vi "Robot Polish Demo.vi"() -> ()   [LabVIEW 2016]
uses:
  <vilib>/Platform/TimedLoop/XDataNode/timing_clust.ctl
  <vilib>/Platform/TimedLoop/XDataNode/nitl_modes.ctl
  <vilib>/Platform/TimedLoop/XDataNode/wakeup.ctl
  Subsystems/Global Variables.vi
  <vilib>/FPGAPlugInAG/PXI-7833R/niLvFpga_Open_PXI-7833R.vi
  <vilib>/Utility/error.llb/Error Cluster From Error Code.vi
  <vilib>/rvi/errors/niLvFpgaAdjustHostInterfaceError.vi
  <vilib>/Utility/file.llb/Write Delimited Spreadsheet (string).vi
  <vilib>/Utility/file.llb/Write Delimited Spreadsheet (DBL).vi
  <vilib>/FPGAPlugInAG/PXI-7833R/niLvFpga_Reset_PXI-7833R.vi
  <vilib>/FPGAPlugInAG/PXI-7833R/niLvFpga_Close_PXI-7833R.vi
  <vilib>/rvi/interface/nirviOpenFPGA/nirviOpenFPGA.xnode
  FPGA Bitfiles/PhantomControlPI_FPGATarget_QuadCtr2_E2412E44.lvbitx
  IRISS_FPGA_IO.vi
  <vilib>/rvi/interface/nirviReadWriteControl/nirviReadWriteControl.xnode
  <vilib>/platform/TimedLoop/XDataNode/XDataNode.xnode
  <vilib>/rvi/interface/nirviMethod/nirviMethod.xnode
  <vilib>/rvi/interface/nirviCloseFPGA/nirviCloseFPGA.xnode
  Library/KevinLibraryAll/labview2011/kevLib2011.lvlib
  NiFpgaLv.dll
  <vilib>/Platform/TimedLoop/XDataNode/XDNodeRunTimeDep.lvlib
panel:
  in  "OCT Z":dbl
  out "Current Iter. No.":u16
  in  "Set Iter. No.":i32=5
  in  "Learning Type":enum8{"Cyber Learning", "Physical Learning"}(ring)=enum."Physical Learning"
  out "RUY Cluster":T1
  in  "Pause":bool caption="To M/S"
  in  "No. Cycles":u8=1
  in  "L4 [deg]":dbl
  in  "L3 [mm]":dbl step=0.1
  in  "L2 [deg]":dbl
  in  "L1 [deg]":dbl
  out "Trajectory Cluster":T2
  out "Update Mdl & Traj":bool=TRUE
  out "Stage PID Cluster":T3={"Stage Z PID"={"Kp"=0.0005, "Kd"=0.001, "Ki"=0.0}, "Stage Y PID"={"Kp"=0.0003, "Kd"=0.01, "Ki"=0.0}, "Stage X PID"={"Kp"=0.0003, "Kd"=0.01, "Ki"=0.0}}
  out "L1 to L4 PID Cluster":T4={"L1 PID Gains"={"Kp"=0.005, "Kd"=0.5, "Ki"=0.0005}, "L2 PID Gains"={"Kp"=0.01, "Kd"=1.0, "Ki"=0.0005}, "L3 PID Gains"={"Kp"=0.05, "Kd"=1.0, "Ki"=0.0005}, "L4 PID Gains"={"Kp"=0.1, "Kd"=1.0, "Ki"=0.0005}}
  in  "IRISS GUI":T5(tab)
  in  "OCT Home Dir":bool
  out "X Stage out [mm] 2":dbl caption="Stage X [mm]" format="%#.4f"
  out "Z Stage out [mm] 2":dbl caption="Stage Z [mm]" format="%#.4f"
  out "Y Stage out [mm] 2":dbl caption="Stage Y [mm]" format="%#.4f"
  out "Vacuum Force [mmHg]  2":i32 caption="[mmHg]"
  out "Finished Late Counts":u16
  out "Emergency alarm":bool
  out "Remote sender engaged":bool
  in  "L2 PID Gains":cluster{"Kp":dbl, "Kd":dbl, "Ki":dbl}={"Kp"=0.01, "Kd"=1.0, "Ki"=0.005}
  in  "L3 PID Gains":cluster{"Kp":dbl, "Kd":dbl, "Ki":dbl}={"Kp"=0.05, "Kd"=1.0, "Ki"=0.0005}
  in  "L4 PID Gains":cluster{"Kp":dbl, "Kd":dbl, "Ki":dbl}={"Kp"=0.1, "Kd"=0.1, "Ki"=0.0005}
  in  "L1 PID Gains":cluster{"Kp":dbl, "Kd":dbl, "Ki":dbl}={"Kp"=0.01, "Kd"=0.5, "Ki"=0.001}
  out "Current System State":T6(ring)
  out "State changing":bool
  out "Tip out Posit":dbl[](array[numeric]) caption="Position [mm]" format="%#.3f"
  out "Tip cmd Posit":dbl[](array[numeric]) caption="Command [mm]" format="%#.3f"
  out "L4 out Posit":dbl caption="y [deg]" format="%#.2g"
  out "L4 cmd Posit":dbl caption="r [deg]" format="%#.2g"
  out "L3 out Posit":dbl caption="y [mm]" format="%#.2g"
  out "L3 cmd Posit":dbl caption="r [mm]" format="%#.2g"
  out "L2 out Posit":dbl caption="y [deg]" format="%#.2g"
  out "L2 cmd Posit":dbl caption="r [deg]" format="%#.2g"
  out "L1 out Posit":dbl caption="y [deg]" format="%#.2g"
  out "L1 cmd Posit":dbl caption="r [deg]" format="%#.2g"
  out "State Flag Array":bool[](array[boolean])
  out "Irrigation Engaged? 2":bool caption="Irrigation Engaged"
  out "Task Space Error":dbl[][](graph)
  in  "Learning Gains":dbl[](array[numeric])=[0.75, 1.0, 0.75, 0.0]
  in  "Joint Limits":dbl[][](array[numeric])=[[-8.0, 50.0], [-35.0, 35.0], [-5.0, 20.0], [-180.0, 180.0]] format="%#.3g"
  out "First Trk Pt":dbl[](array[numeric]) format="%#.3g"
  in  "Offset Home 2 RCM":dbl[](array[numeric])=[-7.7, 37.0, 55.0, 0.0] format="%#.3g"
  out "Error(s) Out on Program End":errorcluster
  out "L4 Chart":dbl(graph)
  out "L3 Chart":dbl(graph)
  out "L2 Chart":dbl(graph)
  out "L1 Chart":dbl(graph)
  out "L1 Tracking":dbl[][](graph)
  out "L2 Tracking":dbl[][](graph)
  out "L3 Tracking":dbl[][](graph)
  out "L4 Tracking":dbl[][](graph)
  out "L1 Cmd":dbl[](graph)
  out "L2 Cmd":dbl[](graph)
  out "L4 Cmd":dbl[](graph)
  out "L3 Cmd":dbl[](graph)
  in  "Clear Charts":bool
  out "AC Pressure [mmHg]":sgl
  in  "Irrigation?":bool
  in  "PID ON/OFF":bool
  in  "Vac PID Gains":cluster{"Kp":dbl, "Kd":dbl, "Ki":dbl, "Ts":dbl}={"Kp"=5.0, "Kd"=0.0, "Ki"=5.0, "Ts"=0.01}
  in  "Vac Cmd":sgl min=0 max=100 step=1 format="%#_13g"
  in  "Target IOP":sgl=20.0 min=0 max=100 step=1 format="%#_13g"
  out "IOP Ctrl":T7(graph)
  out "Pressure Sensors":T8(graph)
  in  "Remote Control Source":u16(ring) caption="Remote Source" items=["Surgical Console", "Joystick"]
  in  "Reset Joystick":bool caption="Encoder Reset"
  in  "Max Limit [mmHg]":dbl=600.0
  out "Pressure Reading":dbl[](array[numeric]) caption="IOP Output [mmHg]"
  in  "Hydration":bool
  out "Vac Input":sgl
  in  "Wait Time [ms]":i32=200
  in  "Vac Step Size":sgl=50.0 min=0 max=100 step=1 format="%#_13g"
  in  "Increase":bool
  in  "Vacuum Step":bool
  in  "Take IOP Data":bool
  out "Elaspsed Time":sgl
  in  "Seconds of Data":sgl=5.0
  out "File Exists":bool
  out "File Path":path=path "C:/IOPData1.txt"
  in  "Data No":i16=1 min=1 step=1
  in  "Eye No":i16=1 min=1 step=1
  out "OCT Z out [mm]":dbl caption="OCT Out Z [mm]" format="%#.4f"
  out "OCT Z cmd [mm]":dbl=6.0 caption="OCT Z Ref [mm]" min=0.0 max=12.0 step=0.5
  in  "OCT Z PID Gains":cluster{"Kp":dbl, "Kd":dbl, "Ki":dbl}={"Kp"=0.0003, "Kd"=0.0001, "Ki"=0.01}
  out "Z Stage out [mm]":dbl caption="Output Z [mm]" format="%#.4f"
  out "Z Stage cmd [mm]":dbl=6.0 caption="Reference Z [mm]" min=0.0 max=12.0 step=0.5
  out "Y Stage out [mm]":dbl caption="Output Y [mm]" format="%#.4f"
  out "Y Stage cmd [mm]":dbl=6.0 caption="Reference Y  [mm]" min=0.0 max=12.0 step=0.5
  out "X Stage out [mm]":dbl caption="Output X [mm]" format="%#.4f"
  out "X Stage cmd [mm]":dbl=6.0 caption="Reference X [mm]" min=0.0 max=12.0 step=0.5
  in  "Stage Z PID Gains":cluster{"Kp":dbl, "Kd":dbl, "Ki":dbl}={"Kp"=0.0005, "Kd"=0.001, "Ki"=0.0}
  in  "Stage Y PID Gains":cluster{"Kp":dbl, "Kd":dbl, "Ki":dbl}={"Kp"=0.0001, "Kd"=0.005, "Ki"=0.0}
  in  "Stage X PID Gains":cluster{"Kp":dbl, "Kd":dbl, "Ki":dbl}={"Kp"=0.0003, "Kd"=0.01, "Ki"=0.0}
  out "Irrigation Engaged?":bool
  out "Accurus Button":bool[](array[boolean]) caption="Remote Button Command"
  in  "Control: Vacuum Force":i8(slide) min=0 max=78 step=1 scale=0.0..78.0
  out "Voltage Output Ch. B":dbl(graph)
  out "Voltage Output Ch. A":dbl(graph)
  out "Accurus Engaged?":bool
  out "Vacuum Force [mmHg]":i32
  in  "Load Traj":bool caption="To M/S"
  in  "Retract":bool caption="To M/S"
  in  "Stop Accurus":bool caption="To M/S"
  in  "L3 Go Home":bool caption="To M/S"
  in  "Track":bool caption="To M/S"
  in  "Program Stop":bool
  in  "Iterate":bool caption="To M/S"
  # "Track Params"
  # "ILC Params"
  # "Tool Tip Location"
  # "L1"
  # "Robot Status"
  # "X\nY\nZ"
  # "X\nY\nZ"
  # "L2"
  # "System Progress"
  # "L3"
  # "Homing finished"
  # "Task Space Error"
  # "M/S initialization finished"
  # "Trajecoty loading finished"
  # "Tracking initialization finished"
  # "L4"
  # "In Tracking"
  # "Notes: \n2. check state transition\n4. preview trajectory?"
  # "Vacuum"
  # "Calibration"
  # "Space Deform Parameters"
  # "Joint Motion"
  # "S"
  # "L1"
  # "[deg]"
  # "R"
  # "[deg]"
  # "L2"
  # "[deg]"
  # "T"
  # "[mm]"
  # "L3"
  # "[mm]"
  # "L4"
  # "[deg]"
  # "AC & PC Gap"
  # "First Track Point"
  # "L1"
  # "[deg]"
  # "L2"
  # "[deg]"
  # "L3"
  # "[mm]"
  # "L4"
  # "[deg]"
  # "Tracking Joint Limits"
  # "Error Message"
  # "Incision"
  # "Min."
  # "Max."
  # "L1"
  # "L1"
  # "[deg]"
  # "L2"
  # "L2"
  # "[deg]"
  # "L3"
  # "L3"
  # "[mm]"
  # "L4"
  # "L4"
  # "[deg]"
  # "IOP Feedback Control"
  # "Data Saving"
  # "Vacuum Step"
  # "XYZ Stage Control"
  # "OCT Z-Axis"
  # "Foot Pedal Buttons"
  # "Irrigation and Aspiration"
  # "Button 1"
  # "Button 2"
  # "Button 3"
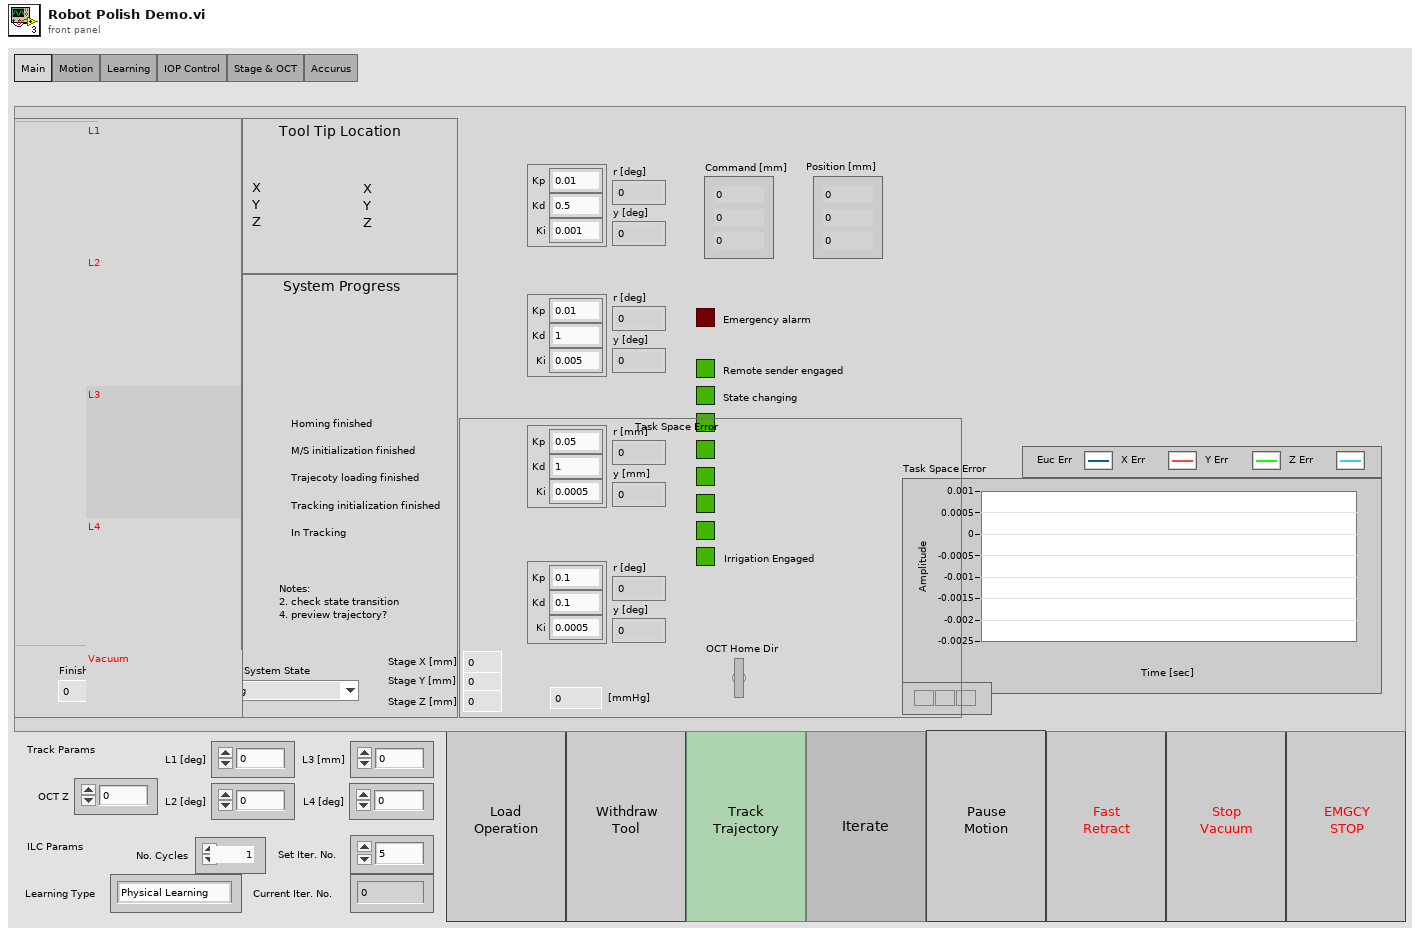
[diagram p1: front panel]
types:
  T1 = cluster{"Ref":cluster{"theta 1 Array":dbl[], "theta 2 Array":dbl[], "d3 Array":dbl[], "theta 4 Array":dbl[]}, "uFF":cluster{"theta 1 Array":dbl[], "theta 2 Array":dbl[], "d3 Array":dbl[], "theta 4 Array":dbl[]}, "yOut":cluster{"theta 1 Array":dbl[], "theta 2 Array":dbl[], "d3 Array":dbl[], "theta 4 Array":dbl[]}}
  T2 = cluster{"Traj Px Array":dbl[], "Traj Py Array":dbl[], "Traj Pz Array":dbl[]}
  T3 = cluster{"Stage Z PID":cluster{"Kp":dbl, "Kd":dbl, "Ki":dbl}, "Stage Y PID":cluster{"Kp":dbl, "Kd":dbl, "Ki":dbl}, "Stage X PID":cluster{"Kp":dbl, "Kd":dbl, "Ki":dbl}}
  T4 = cluster{"L1 PID Gains":cluster{"Kp":dbl, "Kd":dbl, "Ki":dbl}, "L2 PID Gains":cluster{"Kp":dbl, "Kd":dbl, "Ki":dbl}, "L3 PID Gains":cluster{"Kp":dbl, "Kd":dbl, "Ki":dbl}, "L4 PID Gains":cluster{"Kp":dbl, "Kd":dbl, "Ki":dbl}}
  T5 = enum32{"Main", "Motion", "Learning", "IOP Control", "Stage & OCT", "Accurus"}
  T6 = enum16{"Homing", "M/S Initialization", "M/S Operation", "Trajectory Loading", "Tracking Initialization", "Tracking", "Physical Learning", "Cyber Learning"}
  T7 = cluster{"[0]":sgl, "[1]":sgl, "[2]":sgl, "[3]":sgl, "[4]":sgl, "[5]":sgl, "[6]":sgl, "[7]":sgl, "[8]":sgl}
  T8 = cluster{"pressure sensors[0]":sgl, "pressure sensors[1]":sgl, "pressure sensors[2]":sgl, "pressure sensors[3]":sgl, "pressure sensors[4]":sgl, "pressure sensors[5]":sgl, "pressure sensors[6]":sgl, "pressure sensors[7]":sgl, "pressure sensors[8]":sgl}
  T9 = cluster{"theta 1 Array":dbl[], "theta 2 Array":dbl[], "d3 Array":dbl[], "theta 4 Array":dbl[]}
  T10 = cluster{"Prev L1 to L4 Posit":dbl[], "Prev Stage Posit":dbl[], "Prev OCT Z Posit":dbl}
  T11 = typedef "XDNodeRunTimeDep.lvlib/timing_clust.ctl" = cluster{"Expected End [f-1]":u64, "Actual End [f-1]":u64, "Finished Late? [f-1]":bool, "Expected End [i-1]":u64, "Actual End [i-1]":u64, "Finished Late? [i-1]":bool, "Expected Start [i]":u64, "Actual Start [i]":u64, "Expected Start [f]":u64, "Actual Start [f]":u64, "Source Name":string, "Structure Name":string, "Period":i64, "Deadline":i64, "Offset":i64, "Start":i64, "Priority":i32, "Timeout":i32, "Mode":T12, "Wakeup Reason":T13, "Error":errorcluster, "Source Type":string, "Secondary Source Type":string, "Global End Time":u64, "Global Start Time":u64, "Frame Duration":u64, "Iteration Duration":u64, "Assigned CPU":i32, "I/O Scan Engine Mode":u32}
  T12 = typedef "XDNodeRunTimeDep.lvlib/nitl_modes.ctl" = enum32{"No Change", "Process missed periods, maintain original phase", "Discard missed periods, maintain original phase", "Process missed periods, ignore original phase", "Discard missed periods, ignore original phase"}
  T13 = typedef "XDNodeRunTimeDep.lvlib/wakeup.ctl" = enum32{"Normal", "Aborted", "Asynchronous wakeup", "Timing source error", "Timed loop error", "Timeout"}
  T14 = cluster{"L1 to L4 PID Cluster":cluster{"L1 PID Gains":cluster{"Kp":dbl, "Kd":dbl, "Ki":dbl}, "L2 PID Gains":cluster{"Kp":dbl, "Kd":dbl, "Ki":dbl}, "L3 PID Gains":cluster{"Kp":dbl, "Kd":dbl, "Ki":dbl}, "L4 PID Gains":cluster{"Kp":dbl, "Kd":dbl, "Ki":dbl}}, "Stage PID Cluster":cluster{"Stage Z PID":cluster{"Kp":dbl, "Kd":dbl, "Ki":dbl}, "Stage Y PID":cluster{"Kp":dbl, "Kd":dbl, "Ki":dbl}, "Stage X PID":cluster{"Kp":dbl, "Kd":dbl, "Ki":dbl}}, "OCT Z PID Gains":cluster{"Kp":dbl, "Kd":dbl, "Ki":dbl}}
  T15 = enum8{"Enabled", "Disabled", "Disabled and Grayed Out"}
  T16 = cluster{"Accurus button":bool[], "Accurus engaged?":bool, "Vacuum Force":i32, "Accurus Ch. A Vout":dbl, "Accurus Ch. B Vout":dbl, "Irrigation engaged?":bool}
  T17 = cluster{"pressure sensors[0]":sgl, "pressure sensors[1]":sgl, "pressure sensors[2]":sgl, "pressure sensors[3]":sgl, "pressure sensors[4]":sgl, "pressure sensors[5]":sgl, "pressure sensors[6]":sgl, "pressure sensors[7]":sgl, "pressure sensors[8]":sgl}[]
  T18 = cluster{"Last L1 to L4 Posit":dbl[], "Last Stage Posit":dbl[], "Last OCT Z Posit":dbl}
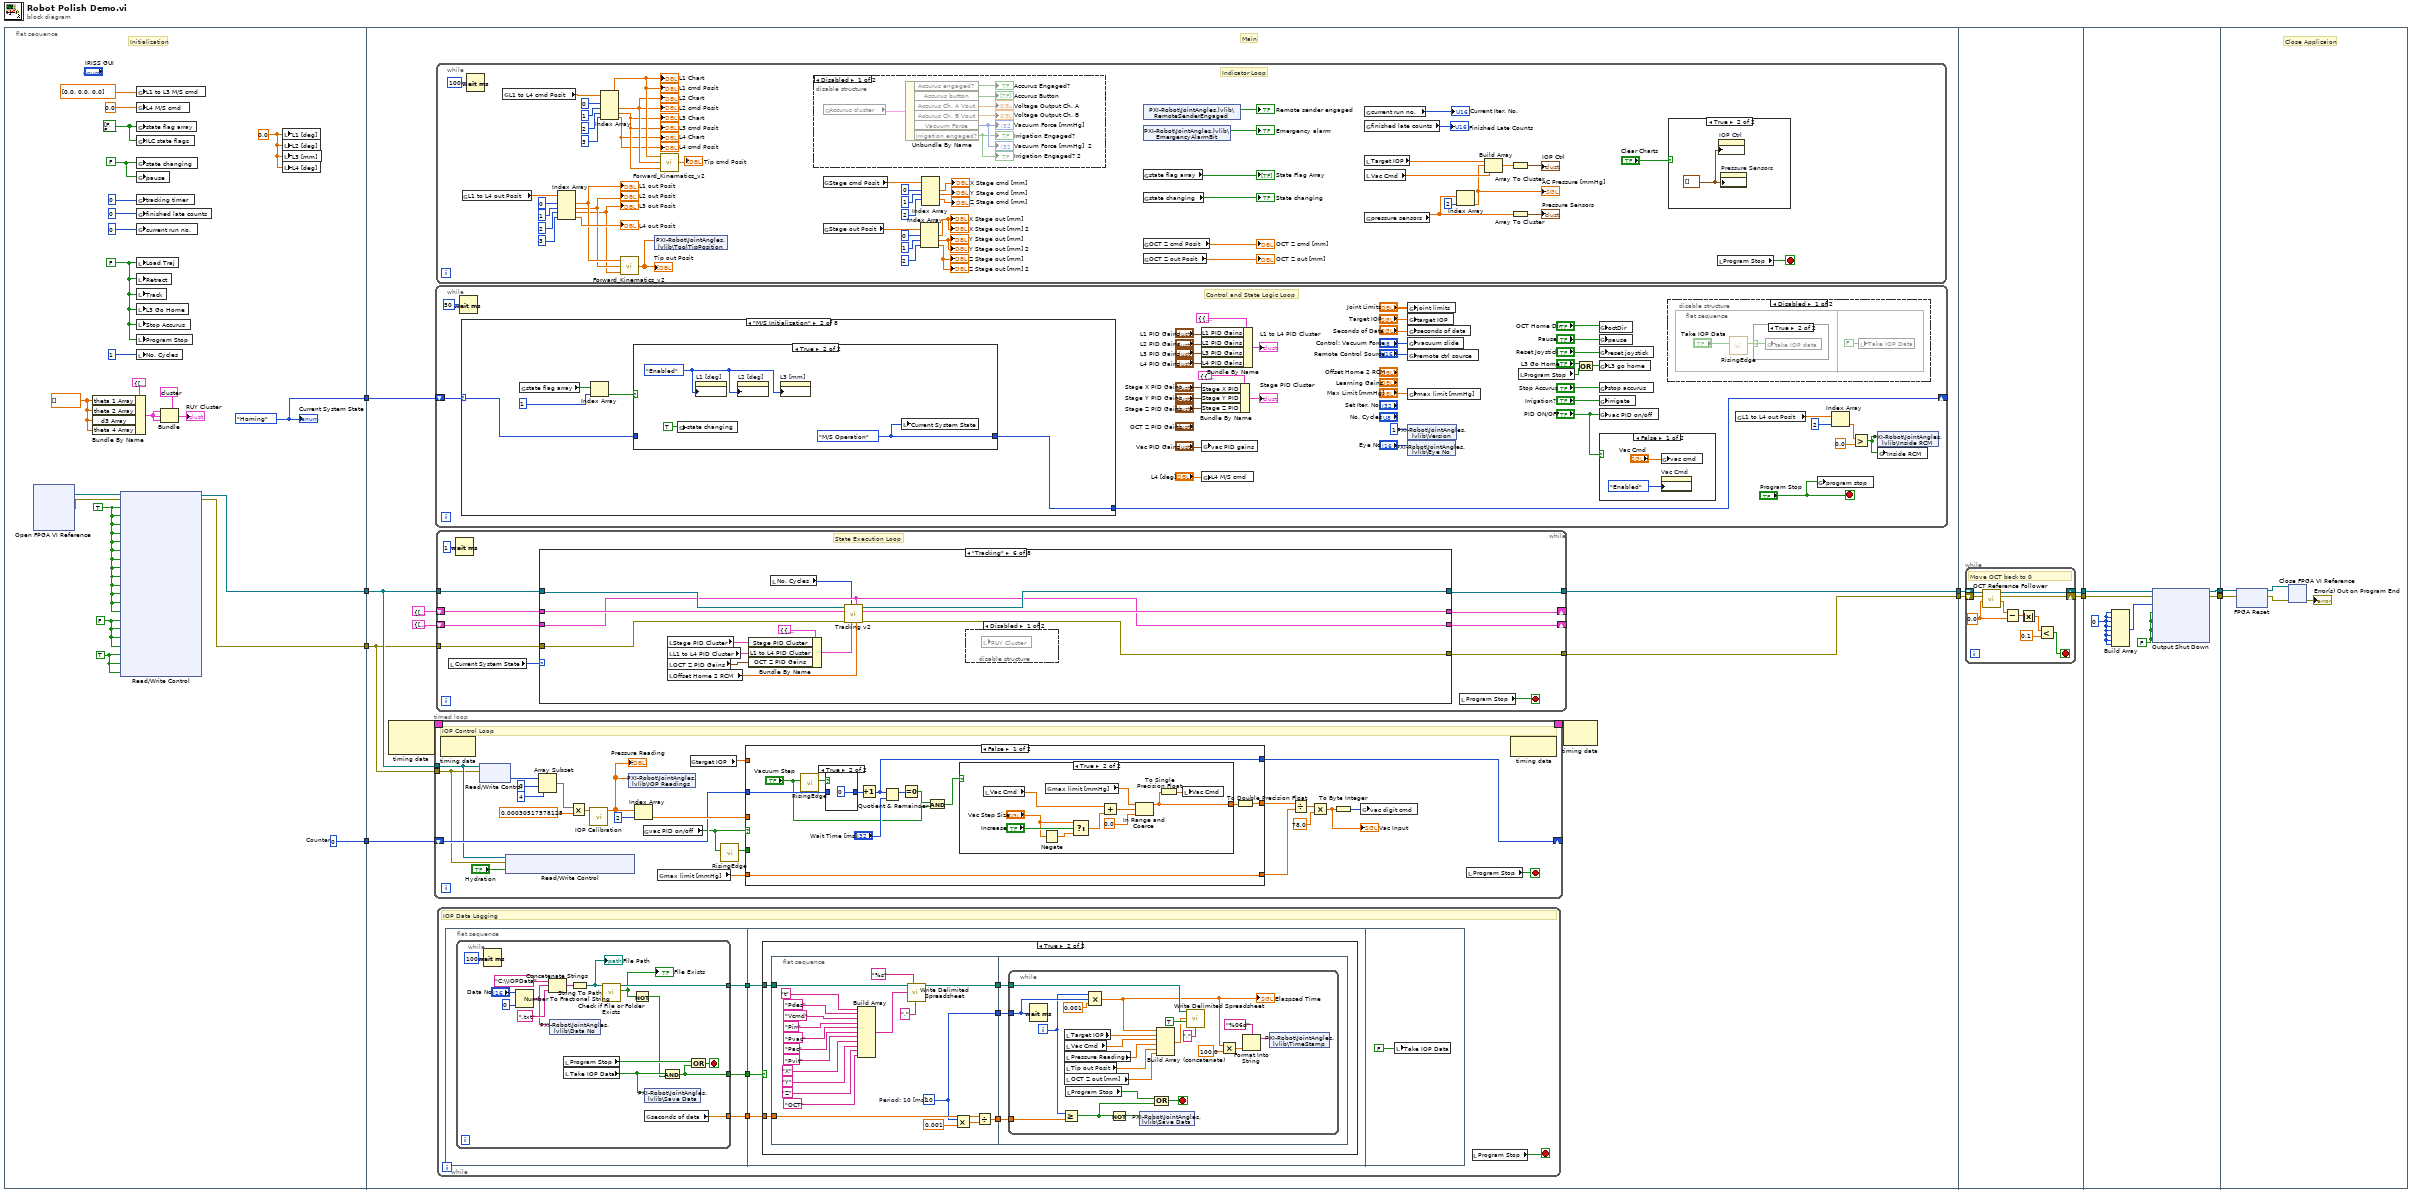
[diagram p0: block diagram]
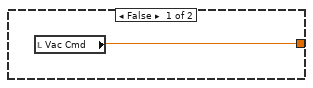
[diagram p4: hidden frame]
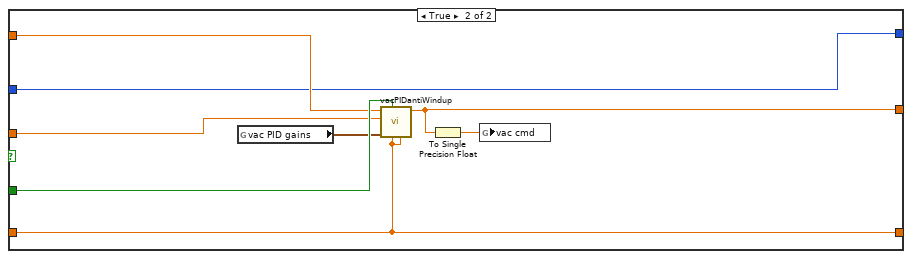
[diagram p5: hidden frame]
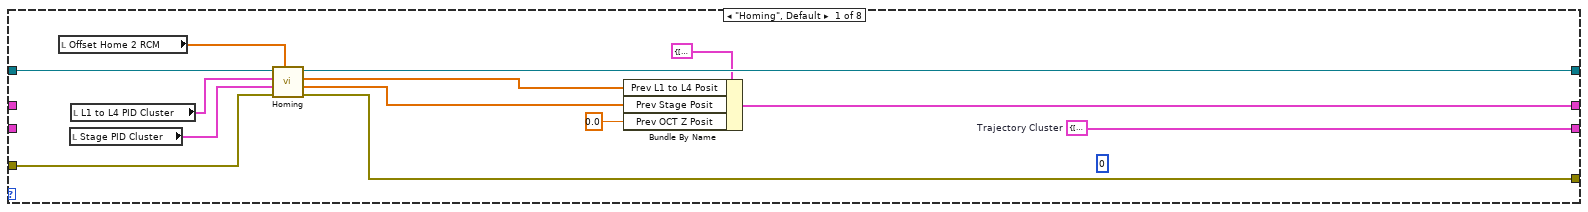
[diagram p8: hidden frame]
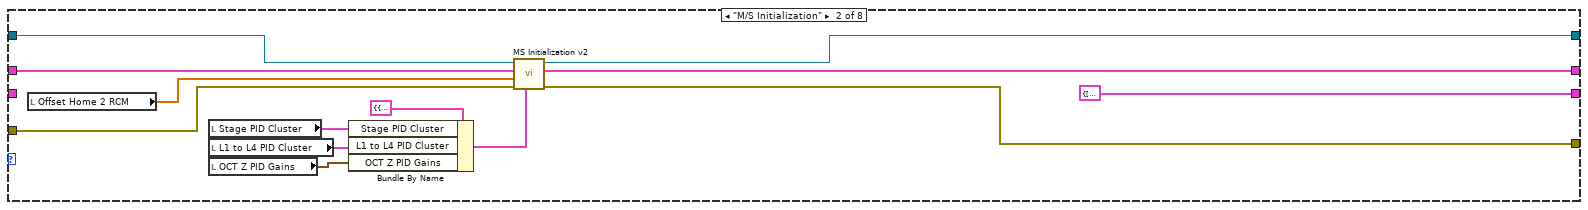
[diagram p9: hidden frame]
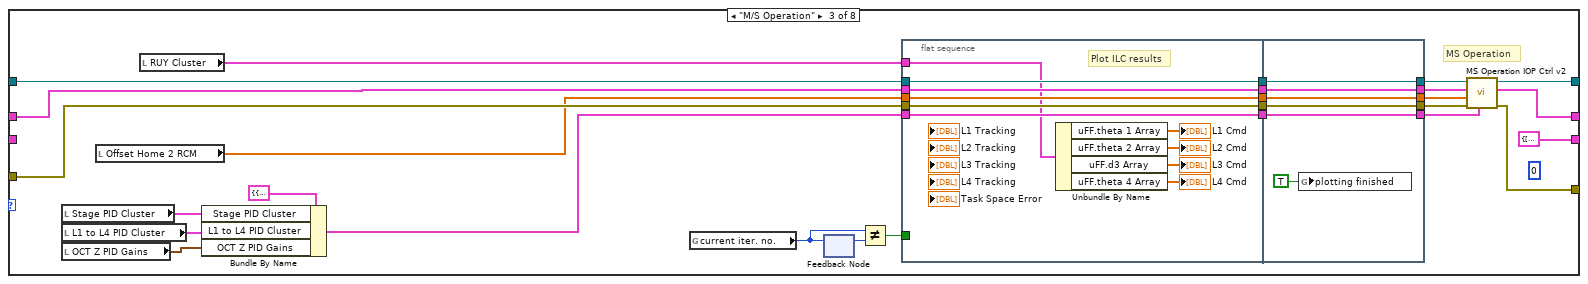
[diagram p10: hidden frame]
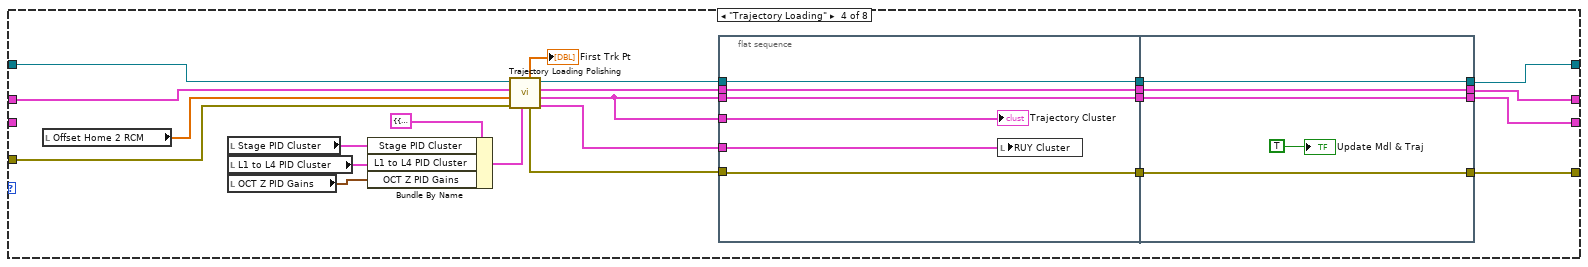
[diagram p11: hidden frame]
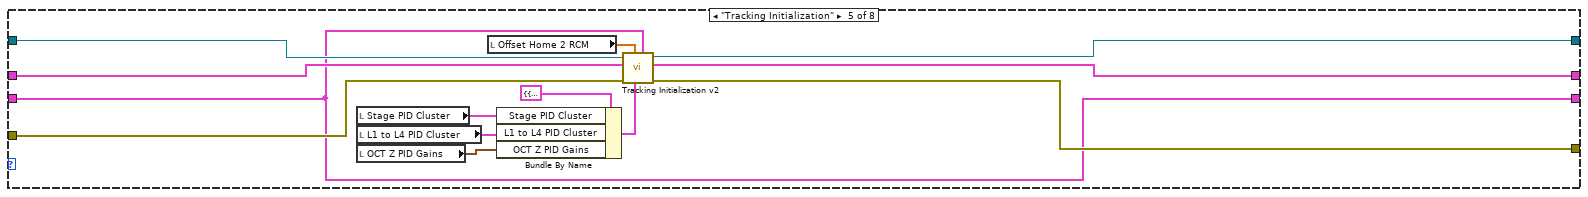
[diagram p12: hidden frame]
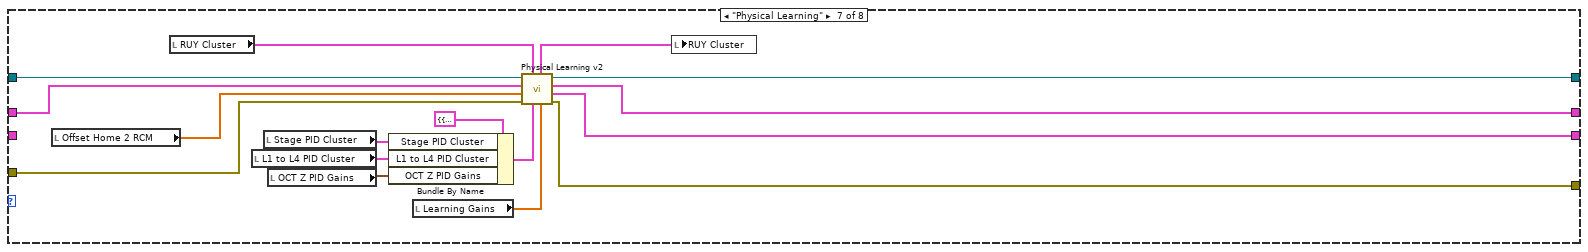
[diagram p14: hidden frame]
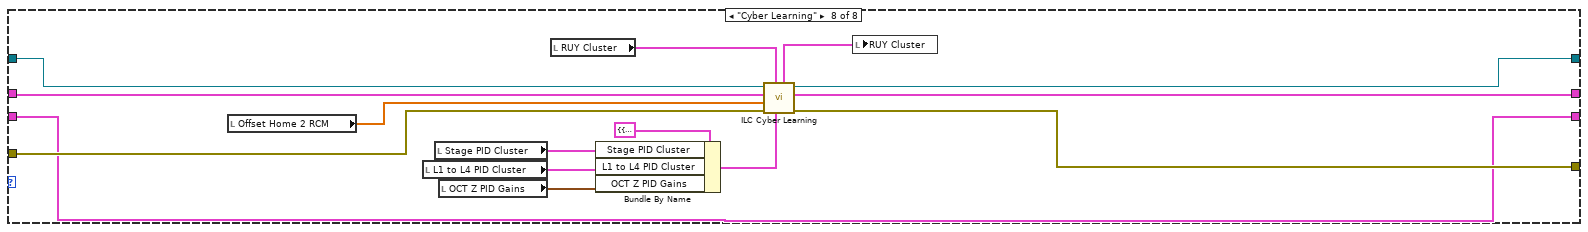
[diagram p15: hidden frame]
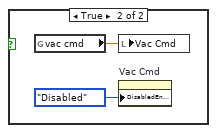
[diagram p18: hidden frame]
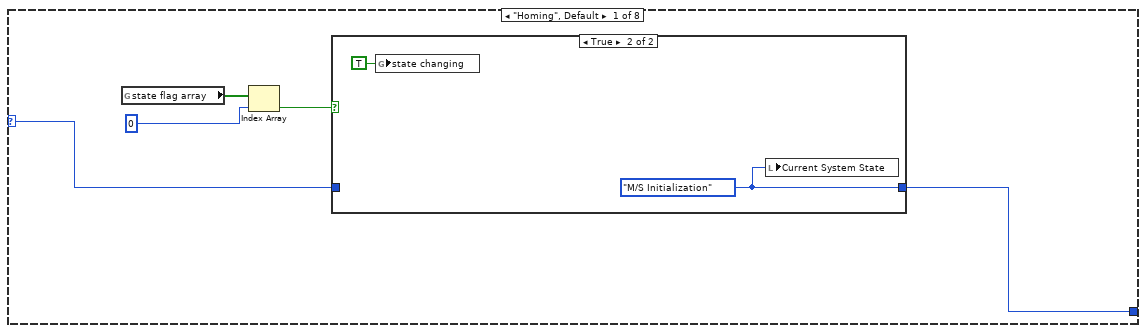
[diagram p19: hidden frame]
diagram:
  n1 = flat-sequence {
    tunnel: [w29] -> w10
    tunnel: [w28] -> w9
    tunnel: [w24] -> w8
    tunnel: [w11] -> w7
    tunnel: w7 -> [w38]
    tunnel: w8 -> [w41]
    tunnel: w9 -> [w39]
    tunnel: w10 -> [w37]
    tunnel: [w36] -> w4
    tunnel: [w35] -> w2
    tunnel: w4 -> [w608]
    tunnel: [w610] -> w3
    tunnel: w2 -> [w609]
    tunnel: [w611] -> w1
    tunnel: [w625] -> w6
    tunnel: [w624] -> w5
    tunnel: w3 -> [w622]
    tunnel: w1 -> [w623]
    tunnel: w6 -> [w630]
    tunnel: w5 -> [w629]
    frame #0 {
      w11 = 0  # Counter
      w12 = dbl[] [] ("theta 1 Array")
      w18 = 0.0 ("L4 M/S cmd")
      w24 = T6."Homing" ("Current State")
      w17 = bool[] [FALSE, FALSE, FALSE, FALSE, FALSE, FALSE, FALSE, FALSE, FALSE] ("state flag array")
      w25 = FALSE ("state changing")
      w33 = TRUE ("Conn0/DIO12 Button 1")
      w32 = FALSE ("Reset")
      w34 = TRUE ("Reset")
      w26 = FALSE ("program stop")
      # "Initialization"
      n2 = xnode "Open FPGA VI Reference"() -> ("FPGA VI Reference Out"=w31:refnum<k20>, "error out"=w30:errorcluster)  [unwired: 2 in]
      n3 = Bundle By Name(cluster=T9 {"theta 1 Array"=[], "theta 2 Array"=[], "d3 Array"=[], "theta 4 Array"=[]} ("uFF"), "theta 1 Array"=w12, "theta 2 Array"=w12, "d3 Array"=w12, "theta 4 Array"=w12) -> (w13:T9)
      n4 = xnode "Read/Write Control"("FPGA VI Reference In"=w31, "error in"=w30, "Reset 1"=w34, "Reset 3"=w34, "Reset 9"=w34, "Reset 10"=w34, "Reset 11"=w34, "Reset 12"=w34, "Reset 13"=w34, "Reset 14"=w34, "Reset 15"=w34, "Reset 16"=w34, "Reset 17"=w34, "Reset C1-1"=w34, "Reset C1-4"=w34, "INHB X"=w32, "INHB Y"=w32, "INHB Z"=w32, "INHB OCT Mot"=w32, "Conn0/DIO12 Button 1"=w33, "Conn0/DIO13 Button 2"=w33, "Conn0/DIO15 Button 4"=w33) -> ("FPGA VI Reference Out"=w28:refnum<k20>, "error out"=w29:errorcluster)
      n5 = global write "Global Variables.vi" "L1 to L3 M/S cmd"(dbl[] [0.0, 0.0, 0.0] ("L1 to L3 M/S cmd")) -> ()
      n6 = global write "Global Variables.vi" "L4 M/S cmd"(0.0 ("L4 M/S cmd")) -> ()
      n7 = global write "Global Variables.vi" "state flag array"(w17) -> ()
      n8 = global write "Global Variables.vi" "ILC state flags"(w17) -> ()
      n9 = global write "Global Variables.vi" "state changing"(w25) -> ()
      n10 = global write "Global Variables.vi" "pause"(w25) -> ()
      n11 = global write "Global Variables.vi" "tracking timer"(0 ("finished late counts")) -> ()
      n12 = global write "Global Variables.vi" "finished late counts"(u16 0 ("finished late counts")) -> ()
      n13 = global write "Global Variables.vi" "current run no."(u8 0 ("current run no.")) -> ()
      n14 = local write "Load Traj"(w26) -> ()
      n15 = local write "Retract"(w26) -> ()
      n16 = local write "Track"(w26) -> ()
      n17 = local write "L3 Go Home"(w26) -> ()
      n18 = local write "Stop Accurus"(w26) -> ()
      n19 = local write "Program Stop"(w26) -> ()
      n20 = local write "No. Cycles"(1 ("No. Cycles")) -> ()
      n21 = Bundle(cluster=T1 {"Ref"={"theta 1 Array"=array[6000 elements], "theta 2 Array"=array[6000 elements], "d3 Array"=array[6000 elements], "theta 4 Array"=array[6000 elements]}, "uFF"={"theta 1 Array"=array[6000 elements], "theta 2 Array"=array[6000 elements], "d3 Array"=array[6000 elements], "theta 4 Array"=array[6000 elements]}, "yOut"={"theta 1 Array"=[], "theta 2 Array"=[], "d3 Array"=[], "theta 4 Array"=[]}} ("Cluster"), "Ref"=w13, "uFF"=w13, "yOut"=w13) -> (→"RUY Cluster":T1)
      n22 = local write "L1 [deg]"(w18) -> ()
      n23 = local write "L2 [deg]"(w18) -> ()
      n24 = local write "L3 [mm]"(w18) -> ()
      n25 = local write "L4 [deg]"(w18) -> ()
      "Current System State" <- w24
    }
    frame #1 {
      # "Main"
      n26 = node-c288 ("Input Node")() -> (w44:T11)  [unwired: 2 in]
      n27 = timed-loop {
        timing: w44 -> [_]
        timing-out: [_] -> w43
        tunnel: w39 -> [w129]
        tunnel: w37 -> [w128]
        shift-right: [w130] -> _
        shift-left: w38 -> [w131]
        stop <- w139 stop-if-true
        # "IOP Control Loop"
        n28 = node-c288() -> ()  [unwired: 1 in, 1 out]
        n29 = xnode "Read/Write Control"("FPGA VI Reference In"=w129, "error in"=w128) -> ("AI"=w142:i16[])  [unwired: 2 out]
        n30 = xnode "Read/Write Control"("FPGA VI Reference In"=w129, "error in"=w128, "Hydration On/Off (Connector2/DIO28)"="Hydration") -> ()  [unwired: 2 out]
        n31 = Array Subset(array=w142, index=0, length=4) -> (w147:i16[])
        n32 = Multiply(x=w147, y=0.00030517578125) -> (x*y=w134:dbl[])
        n33 = call "IOP Calibration.vi"("IOP Input [V]"=w134) -> ("IOP Output [mmHg]"=w123:dbl[])  [unwired: 10 in]
        "Pressure Reading" <- w123
        n34 = shared-variable "PXI-Robot\\JointAngles.lvlib\\IOP Readings"(w123) -> ()  [unwired: 1 in, 1 out]
        n35 = Index Array(array=w123, index=2) -> (element=w140:dbl)
        n36 = global read "Global Variables.vi" "vac PID on/off"() -> (w124:bool)
        n37 = global read "Global Variables.vi" "max limit [mmHg]"() -> (w125:dbl)
        n38 = global read "Global Variables.vi" "target IOP"() -> (w126:sgl)
        n39 = call "RisingEdge.vi"("Signal In"=w124) -> ("Rising Edge"=w141:bool)  [unwired: 10 in]
        n40 = case shown="False" w124 {
          tunnel: w140 -> [_ w176]
          tunnel: w126 -> [_ w177]
          tunnel: [w159 w180] -> w138
          tunnel: w125 -> [w158 w179]
          tunnel: [w158 w179] -> w132
          tunnel: w141 -> [_ w178]
          tunnel: w131 -> [w151 w175]
          tunnel: [w148 w175] -> w130
          frame False {
            n41 = call "RisingEdge.vi"("Signal In"="Vacuum Step") -> ("Rising Edge"=w152:bool)  [unwired: 10 in]
            n42 = case shown="True" w152 {
              tunnel: [w160 0] -> w155
              tunnel: w151 -> [w160 _]
              frame False {
              }
              frame True {
              }
            }
            n43 = Increment(x=w155) -> (x+1=w148:i32)
            n44 = Quotient & Remainder(x=w148, y="Wait Time [ms]") -> (x-y*floor(x/y)=w154:i32)  [unwired: 1 out]
            n45 = Equal To 0?(x=w154) -> (x = 0?=w156:bool)
            n46 = And(x=w156, y="Vacuum Step") -> (x .and. y?=w150:bool)
            n47 = case shown="True" w150 {
              tunnel: [w162 w172] -> w157
              frame False {
                n48 = local read "Vac Cmd"() -> (w162:sgl)
              }
              frame True {
                n49 = local read "Vac Cmd"() -> (w166:sgl)
                n50 = Negate(x="Vac Step Size") -> (-x=w164:sgl)
                n51 = global read "Global Variables.vi" "max limit [mmHg]"() -> (w163:dbl)
                n52 = Select(t="Vac Step Size", s="Increase", f=w164) -> (s? t:f=w168:sgl)
                n53 = Add(x=w166, y=w168) -> (x+y=w171:sgl)
                n54 = In Range and Coerce(upper limit=w163, x=w171, lower limit=0.0 ("y")) -> (coerced(x)=w172:dbl)  [unwired: 1 out]
                n55 = To Single Precision Float(number=w172) -> (single precision float=w167:sgl)
                n56 = local write "Vac Cmd"(w167) -> ()
              }
            }
            n57 = To Double Precision Float(number=w157) -> (double precision float=w159:dbl)
          }
          frame True {
            n58 = global read "Global Variables.vi" "vac PID gains"() -> (w174:cluster{"Kp":dbl, "Kd":dbl, "Ki":dbl, "Ts":dbl})
            n59 = call "vacPIDantiWindup.vi"("Saturation U"=w179, "Saturation M"=w179, "Reset"=w178, "PID Gains"=w174, "Feedback"=w176, "Reference"=w177) -> ("Control"=w180:dbl)  [unwired: 5 in]
            n60 = To Single Precision Float(number=w180) -> (single precision float=w173:sgl)
            n61 = global write "Global Variables.vi" "vac cmd"(w173) -> ()
          }
        }
        n62 = Divide(x=w138, y=w132) -> (x/y=w137:dbl)
        n63 = Multiply(x=w137, y=78.0) -> (x*y=w133:dbl)
        "Vac Input" <- w133
        n64 = To Byte Integer(number=w133) -> (8bit integer=w135:i8)
        n65 = global write "Global Variables.vi" "vac digit cmd"(w135) -> ()
        n66 = local read "Program Stop"() -> (w139:bool)
        n67 = node-c288() -> ()  [unwired: 1 in, 1 out]
      }
      n68 = while {
        shift-right: [w435] -> _
        shift-left: w41 -> [w436]
        stop <- "Program Stop" stop-if-true
        # "Control and State Logic Loop"
        n69 = Wait (ms)(milliseconds to wait=u32 50) -> ()  [unwired: 1 out]
        n70 = case shown="\"M/S Initialization\"" w436 {
          selector: w436 -> [w467 w473 w488 w543 w553 w560 w587 w599]
          tunnel: [w466 w474 w487 w544 w552 w561 w589 w598] -> w435
          frame "Homing", Default {
            n71 = global read "Global Variables.vi" "state flag array"() -> (w468:bool[])
            n72 = Index Array(array=w468, index=0) -> (element=w465:bool)
            n73 = case shown="True" w465 {
              tunnel: [w470 w471] -> w466
              tunnel: w467 -> [w470 _]
              frame False {
                # "homing in process"
              }
              frame True {
                w471 = T6."M/S Initialization" ("Current State")
                # "finish homing"
                n74 = global write "Global Variables.vi" "state changing"(TRUE ("state changing")) -> ()
                n75 = local write "Current System State"(w471) -> ()
              }
            }
          }
          frame "M/S Initialization" {
            n76 = global read "Global Variables.vi" "state flag array"() -> (w476:bool[])
            n77 = Index Array(array=w476, index=1) -> (element=w475:bool)
            n78 = case shown="True" w475 {
              tunnel: [w478 w479] -> w474
              tunnel: w473 -> [w478 _]
              frame False {
              }
              frame True {
                w479 = T6."M/S Operation" ("Current State")
                w480 = T15."Enabled" ("Disabled")
                n79 = global write "Global Variables.vi" "state changing"(TRUE ("state changing")) -> ()
                n80 = property on="L1 [deg]" class="DigNum (strict)"("DisabledEnum"=w480) -> ()  [unwired: 2 in, 2 out]
                n81 = property on="L2 [deg]" class="DigNum (strict)"("DisabledEnum"=w480) -> ()  [unwired: 2 in, 2 out]
                n82 = property on="L3 [mm]" class="DigNum (strict)"("DisabledEnum"=w480) -> ()  [unwired: 2 in, 2 out]
                n83 = local write "Current System State"(w479) -> ()
              }
            }
          }
          frame "M/S Operation" {
            n84 = Build Array("Load Traj", "Iterate", "Track") -> (w484:bool[])
            n85 = Boolean Array To Number(Boolean array=w484) -> (number=w486:u32)
            n86 = case shown="2" w486 {
              tunnel: w488 -> [w490 w514 w525 _]
              tunnel: [w490 w518 w528 w539] -> w487
              frame 0, Default {
                n87 = shared-variable "PXI-Robot\\JointAngles.lvlib\\RemoteSenderEngaged"() -> (w489:bool)  [unwired: 1 in, 1 out]
                n88 = case shown="False" w489 {
                  frame False {
                    n89 = Build Array("L1 [deg]", "L2 [deg]", "L3 [mm]") -> (w494:dbl[])
                    n90 = global write "Global Variables.vi" "OCT Z cmd Posit"("OCT Z") -> ()
                    n91 = global write "Global Variables.vi" "L1 to L3 M/S cmd"(w494) -> ()
                  }
                  frame True {
                    n92 = shared-variable "PXI-Robot\\JointAngles.lvlib\\Move XYZ"() -> (w496:bool)  [unwired: 1 in, 1 out]
                    n93 = case shown="True" w496 {
                      frame False {
                        n94 = shared-variable "PXI-Robot\\JointAngles.lvlib\\L1 to L4 Cmd"() -> (w503:dbl[])  [unwired: 1 in, 1 out]
                        n95 = Index Array(array=w503) -> (element #1=w501:dbl, element #2=w500:dbl, element #3=w499:dbl, element #4=w502:dbl)  [unwired: 4 in]
                        n96 = Build Array(w501, w500, w499) -> (w498:dbl[])
                        n97 = local write "L1 [deg]"(w501) -> ()
                        n98 = local write "L2 [deg]"(w500) -> ()
                        n99 = local write "L3 [mm]"(w499) -> ()
                        n100 = global write "Global Variables.vi" "L1 to L3 M/S cmd"(w498) -> ()
                        n101 = global write "Global Variables.vi" "L4 M/S cmd"(w502) -> ()
                      }
                      frame True {
                        w507 = 0.0 ("element")
                        n102 = shared-variable "PXI-Robot\\JointAngles.lvlib\\XYZ Cmd"() -> (w513:dbl[])  [unwired: 1 in, 1 out]
                        n103 = Index Array(array=w513) -> (element #1=w512:dbl, element #2=w511:dbl, element #3=w510:dbl)  [unwired: 3 in]
                        n104 = call "Inverse_Kinematics_to_Deg_mm.vi"("pz"=w510, "py"=w511, "px"=w512) -> ("L3 [mm]"=w506:dbl, "L2 [deg]"=w505:dbl, "L1 [deg]"=w504:dbl)
                        n105 = Build Array(w504, w505, w506) -> (w508:dbl[])
                        n106 = Build Array(w504, w505, w506, w507) -> (w509:dbl[])
                        n107 = global write "Global Variables.vi" "L1 to L3 M/S cmd"(w508) -> ()
                        n108 = shared-variable "PXI-Robot\\JointAngles.lvlib\\L1 to L4 Cmd"(w509) -> ()  [unwired: 1 in, 1 out]
                        n109 = global write "Global Variables.vi" "L4 M/S cmd"(w507) -> ()
                      }
                    }
                    n110 = shared-variable "PXI-Robot\\JointAngles.lvlib\\OCT z command"() -> (w497:dbl)  [unwired: 1 in, 1 out]
                    n111 = local write "OCT Z"(w497) -> ()
                  }
                }
              }
              frame 1 {
                n112 = global read "Global Variables.vi" "current iter. no."() -> (w517:u16)
                n113 = Equal?(x=w517, y=u16 0) -> (x = y?=w516:bool)
                n114 = case shown="True" w516 {
                  tunnel: [w519 w520] -> w518
                  tunnel: w514 -> [w519 _]
                  frame False {
                  }
                  frame True {
                    w520 = T6."Trajectory Loading" ("Current State")
                    w521 = T15."Disabled and Grayed Out" ("Disabled")
                    n115 = global write "Global Variables.vi" "state changing"(TRUE ("state changing")) -> ()
                    n116 = local write "Load Traj"(FALSE ("Load Traj")) -> ()
                    n117 = property on="L1 [deg]" class="DigNum (strict)"("DisabledEnum"=w521) -> ()  [unwired: 2 in, 2 out]
                    n118 = property on="L2 [deg]" class="DigNum (strict)"("DisabledEnum"=w521) -> ()  [unwired: 2 in, 2 out]
                    n119 = local write "Current System State"(w520) -> ()
                    n120 = property on="L3 [mm]" class="DigNum (strict)"("DisabledEnum"=w521) -> ()  [unwired: 2 in, 2 out]
                  }
                }
              }
              frame 2 {
                n121 = global read "Global Variables.vi" "current iter. no."() -> (w527:u16)
                n122 = local read "Set Iter. No."() -> (w526:i32)
                n123 = Greater?(x=w526, y=w527) -> (0:w524:bool)
                n124 = case shown="True" w524 {
                  tunnel: [w529 w530] -> w528
                  tunnel: w525 -> [w529 _]
                  frame False {
                  }
                  frame True {
                    w537 = T15."Disabled and Grayed Out" ("Disabled")
                    n125 = Number To Boolean Array(number="Learning Type") -> (Boolean array=w535:bool[])
                    n126 = Index Array(array=w535) -> (element=w534:bool)  [unwired: 1 in]
                    n127 = Select(t=T6."Tracking Initialization" ("Current State"), s=w534, f=T6."Cyber Learning" ("Current State")) -> (s? t:f=w530:T6)
                    n128 = property on="L1 [deg]" class="DigNum (strict)"("DisabledEnum"=w537) -> ()  [unwired: 2 in, 2 out]
                    n129 = local write "Current System State"(w530) -> ()
                    n130 = property on="L2 [deg]" class="DigNum (strict)"("DisabledEnum"=w537) -> ()  [unwired: 2 in, 2 out]
                    n131 = global write "Global Variables.vi" "state changing"(TRUE ("state changing")) -> ()
                    n132 = local write "Track"(FALSE ("Iterate")) -> ()
                    n133 = property on="L3 [mm]" class="DigNum (strict)"("DisabledEnum"=w537) -> ()  [unwired: 2 in, 2 out]
                  }
                }
              }
              frame 3 {
                w540 = T15."Disabled and Grayed Out" ("Disabled")
                w539 = T6."Tracking Initialization" ("Current State")
                n134 = global write "Global Variables.vi" "state changing"(TRUE ("state changing")) -> ()
                n135 = local write "Iterate"(FALSE ("Iterate")) -> ()
                n136 = property on="L1 [deg]" class="DigNum (strict)"("DisabledEnum"=w540) -> ()  [unwired: 2 in, 2 out]
                n137 = property on="L2 [deg]" class="DigNum (strict)"("DisabledEnum"=w540) -> ()  [unwired: 2 in, 2 out]
                n138 = local write "Current System State"(w539) -> ()
                n139 = property on="L3 [mm]" class="DigNum (strict)"("DisabledEnum"=w540) -> ()  [unwired: 2 in, 2 out]
              }
            }
          }
          frame "Trajectory Loading" {
            n140 = global read "Global Variables.vi" "state flag array"() -> (w546:bool[])
            n141 = Index Array(array=w546, index=2) -> (element=w545:bool)
            n142 = case shown="True" w545 {
              tunnel: [w548 w550] -> w544
              tunnel: w543 -> [w548 _]
              frame False {
              }
              frame True {
                w549 = T15."Enabled" ("Disabled")
                w550 = T6."Tracking Initialization" ("Current State")
                n143 = global write "Global Variables.vi" "state changing"(TRUE ("state changing")) -> ()
                n144 = local write "Current System State"(w550) -> ()
                n145 = property on="Iterate" class="Bool (strict)"("DisabledEnum"=w549) -> ()  [unwired: 2 in, 2 out]
                n146 = property on="Track" class="Bool (strict)"("DisabledEnum"=w549) -> ()  [unwired: 2 in, 2 out]
              }
            }
          }
          frame "Tracking Initialization" {
            n147 = global read "Global Variables.vi" "state flag array"() -> (w555:bool[])
            n148 = Index Array(array=w555, index=3) -> (element=w554:bool)
            n149 = case shown="True" w554 {
              tunnel: w553 -> [w557 _]
              tunnel: [w557 w558] -> w552
              frame False {
              }
              frame True {
                w558 = T6."Tracking" ("Current State")
                n150 = global write "Global Variables.vi" "state changing"(TRUE ("state changing")) -> ()
                n151 = local write "Current System State"(w558) -> ()
              }
            }
          }
          frame "Tracking" {
            n152 = global read "Global Variables.vi" "state flag array"() -> (w563:bool[])
            n153 = Index Array(array=w563, index=4) -> (element=w562:bool)
            n154 = case shown="True" w562 {
              tunnel: [w565 w568] -> w561
              tunnel: w560 -> [w565 w567]
              frame False {
              }
              frame True {
                n155 = case shown="True" "Retract" {
                  tunnel: [w570 w584] -> w568
                  tunnel: w567 -> [w571 _]
                  frame False {
                    n156 = local read "Iterate"() -> (w569:bool)
                    n157 = case shown="True" w569 {
                      tunnel: [w573 w575] -> w570
                      tunnel: w571 -> [w573 _]
                      frame False {
                        n158 = local write "Track"(FALSE ("Track")) -> ()
                      }
                      frame True {
                        n159 = flat-sequence {
                          tunnel: [w580] -> w574
                          tunnel: [w582] -> w575
                          tunnel: w574 -> [w582]
                          frame #0 {
                            n160 = local read "Set Iter. No."() -> (w579:i32)
                            n161 = global read "Global Variables.vi" "current iter. no."() -> (w578:u16)
                            n162 = Greater?(x=w579, y=w578) -> (0:w581:bool)
                            n163 = Select(t=T6."Physical Learning" ("Current State"), s=w581, f=T6."M/S Initialization" ("Current State")) -> (s? t:f=w580:T6)
                          }
                          frame #1 {
                            n164 = local write "Current System State"(w582) -> ()
                            n165 = global write "Global Variables.vi" "state changing"(TRUE ("state changing")) -> ()
                          }
                        }
                      }
                    }
                  }
                  frame True {
                    w584 = T6."M/S Initialization" ("Current State")
                    n166 = global write "Global Variables.vi" "state changing"(TRUE ("state changing")) -> ()
                    n167 = local write "Retract"(FALSE ("Load Traj")) -> ()
                    n168 = local write "Current System State"(w584) -> ()
                  }
                }
              }
            }
          }
          frame "Physical Learning" {
            n169 = global read "Global Variables.vi" "ILC state flags"() -> (w590:bool[])
            n170 = Index Array(array=w590, index=4) -> (element=w588:bool)
            n171 = case shown="True" w588 {
              tunnel: w587 -> [w592 _]
              tunnel: [w592 w594] -> w589
              frame False {
              }
              frame True {
                w594 = T6."M/S Initialization" ("Current State")
                n172 = global write "Global Variables.vi" "state changing"(TRUE ("state changing")) -> ()
                n173 = local write "Iterate"(FALSE ("Iterate")) -> ()
                n174 = global read "Global Variables.vi" "current iter. no."() -> (w596:u16)
                n175 = Increment(x=w596) -> (x+1=w595:u16)
                n176 = global write "Global Variables.vi" "current iter. no."(w595) -> ()
                n177 = local write "Current System State"(w594) -> ()
              }
            }
          }
          frame "Cyber Learning" {
            n178 = global read "Global Variables.vi" "ILC state flags"() -> (w601:bool[])
            n179 = Index Array(array=w601, index=2) -> (element=w600:bool)
            n180 = case shown="True" w600 {
              tunnel: w599 -> [w603 _]
              tunnel: [w603 w604] -> w598
              frame False {
              }
              frame True {
                w604 = T6."M/S Initialization" ("Current State")
                n181 = global read "Global Variables.vi" "current iter. no."() -> (w607:u16)
                n182 = global write "Global Variables.vi" "state changing"(TRUE ("state changing")) -> ()
                n183 = Increment(x=w607) -> (x+1=w606:u16)
                n184 = global write "Global Variables.vi" "current iter. no."(w606) -> ()
                n185 = local write "Current System State"(w604) -> ()
              }
            }
          }
        }
        n186 = Bundle By Name(cluster=T4 {"L1 PID Gains"={"Kp"=0.005, "Kd"=0.5, "Ki"=0.0005}, "L2 PID Gains"={"Kp"=0.01, "Kd"=1.0, "Ki"=0.0005}, "L3 PID Gains"={"Kp"=0.05, "Kd"=1.0, "Ki"=0.0005}, "L4 PID Gains"={"Kp"=0.1, "Kd"=1.0, "Ki"=0.0005}} ("L1 to L4 PID Cluster 2"), "L1 PID Gains"="L1 PID Gains", "L2 PID Gains"="L2 PID Gains", "L3 PID Gains"="L3 PID Gains", "L4 PID Gains"="L4 PID Gains") -> (→"L1 to L4 PID Cluster":T4)
        n187 = Bundle By Name(cluster=T3 {"Stage Z PID"={"Kp"=0.0005, "Kd"=0.001, "Ki"=0.0}, "Stage Y PID"={"Kp"=0.0003, "Kd"=0.01, "Ki"=0.0}, "Stage X PID"={"Kp"=0.0003, "Kd"=0.01, "Ki"=0.0}} ("Stage PID Cluster 2"), "Stage X PID"="Stage X PID Gains", "Stage Y PID"="Stage Y PID Gains", "Stage Z PID"="Stage Z PID Gains") -> (→"Stage PID Cluster":T3)
        n188 = global write "Global Variables.vi" "vac PID gains"("Vac PID Gains") -> ()
        n189 = global write "Global Variables.vi" "L4 M/S cmd"("L4 [deg]") -> ()
        n190 = global write "Global Variables.vi" "joint limits"("Joint Limits") -> ()
        n191 = global write "Global Variables.vi" "target IOP"("Target IOP") -> ()
        n192 = global write "Global Variables.vi" "seconds of data"("Seconds of Data") -> ()
        n193 = global write "Global Variables.vi" "vacuum slide"("Control: Vacuum Force") -> ()
        n194 = global write "Global Variables.vi" "remote ctrl source"("Remote Control Source") -> ()
        n195 = global write "Global Variables.vi" "max limit [mmHg]"("Max Limit [mmHg]") -> ()
        n196 = shared-variable "PXI-Robot\\JointAngles.lvlib\\Version"(i16 1 ("Version")) -> ()  [unwired: 1 in, 1 out]
        n197 = shared-variable "PXI-Robot\\JointAngles.lvlib\\Eye No"("Eye No") -> ()  [unwired: 1 in, 1 out]
        n198 = local read "Program Stop"() -> (w438:bool)
        n199 = Or(x="L3 Go Home", y=w438) -> (x .or. y?=w439:bool)
        n200 = global write "Global Variables.vi" "octDir"("OCT Home Dir") -> ()
        n201 = global write "Global Variables.vi" "pause"("Pause") -> ()
        n202 = global write "Global Variables.vi" "reset joystick"("Reset Joystick") -> ()
        n203 = global write "Global Variables.vi" "L3 go home"(w439) -> ()
        n204 = global write "Global Variables.vi" "stop accurus"("Stop Accurus") -> ()
        n205 = global write "Global Variables.vi" "irrigate"("Irrigation?") -> ()
        n206 = global write "Global Variables.vi" "vac PID on/off"("PID ON/OFF") -> ()
        n207 = case shown="False" "PID ON/OFF" {
          frame False {
            n208 = global write "Global Variables.vi" "vac cmd"("Vac Cmd") -> ()
            n209 = property on="Vac Cmd" class="DigNum (strict)"("DisabledEnum"=T15."Enabled" ("Disabled")) -> ()  [unwired: 2 in, 2 out]
          }
          frame True {
            n210 = global read "Global Variables.vi" "vac cmd"() -> (w464:sgl)
            n211 = local write "Vac Cmd"(w464) -> ()
            n212 = property on="Vac Cmd" class="DigNum (strict)"("DisabledEnum"=T15."Disabled" ("Disabled")) -> ()  [unwired: 2 in, 2 out]
          }
        }
        n213 = disable-structure shown="Disabled" {
          frame Disabled {
            n214 = flat-sequence {
              frame #0 {
                n215 = call "RisingEdge.vi"("Signal In"="Take IOP Data") -> ("Rising Edge"=w457:bool)  [unwired: 10 in]
                n216 = case shown="True" w457 {
                  selector: w457 -> [_ w459]
                  frame False {
                  }
                  frame True {
                    n217 = global write "Global Variables.vi" "take IOP data"(w459) -> ()
                  }
                }
              }
              frame #1 {
                n218 = local write "Take IOP Data"(FALSE ("Take IOP Data")) -> ()
              }
            }
          }
          frame Enabled {
          }
        }
        n219 = global read "Global Variables.vi" "L1 to L4 out Posit"() -> (w424:dbl[])
        n220 = global write "Global Variables.vi" "program stop"("Program Stop") -> ()
        n221 = Index Array(array=w424, index=2) -> (element=w423:dbl)
        n222 = Greater?(x=w423, y=0.0) -> (0:w421:bool)
        n223 = shared-variable "PXI-Robot\\JointAngles.lvlib\\Inside RCM"(w421) -> ()  [unwired: 1 in, 1 out]
        n224 = global write "Global Variables.vi" "Inside RCM"(w421) -> ()
      }
      n225 = while {
        stop <- w218 stop-if-true
        # "Indicator Loop"
        n226 = global read "Global Variables.vi" "L1 to L4 out Posit"() -> (w214:dbl[])
        n227 = Wait (ms)(milliseconds to wait=u32 100) -> ()  [unwired: 1 out]
        n228 = global read "Global Variables.vi" "L1 to L4 cmd Posit"() -> (w211:dbl[])
        n229 = Index Array(array=w214, index #1=0 ("index"), index #2=1 ("index"), index #3=2 ("index"), index #4=3 ("index")) -> (element #1=w216:dbl, element #2=w215:dbl, element #3=w185:dbl, element #4=→"L4 out Posit":dbl)
        "L3 out Posit" <- w185
        "L2 out Posit" <- w215
        "L1 out Posit" <- w216
        n230 = Index Array(array=w211, index #1=0 ("index"), index #2=1 ("index"), index #3=2 ("index"), index #4=3 ("index")) -> (element #1=w190:dbl, element #2=w189:dbl, element #3=w188:dbl, element #4=→"L4 cmd Posit" →"L4 Chart":dbl)
        "L1 cmd Posit" <- w190
        "L3 cmd Posit" <- w188
        "L2 cmd Posit" <- w189
        "L2 Chart" <- w189
        "L1 Chart" <- w190
        "L3 Chart" <- w188
        n231 = call "Forward_Kinematics_v2.vi"("theta 3"=w185, "theta 2"=w215, "theta 1"=w216) -> ("position"=w206:dbl[])
        "Tip out Posit" <- w206
        n232 = shared-variable "PXI-Robot\\JointAngles.lvlib\\ToolTipPosition"(w206) -> ()  [unwired: 1 in, 1 out]
        n233 = call "Forward_Kinematics_v2.vi"("theta 3"=w188, "theta 2"=w189, "theta 1"=w190) -> ("position"=→"Tip cmd Posit":dbl[])
        n234 = disable-structure shown="Disabled" {
          frame Disabled {
            n235 = global read "Global Variables.vi" "Accurus cluster"() -> (w244:T16)
            n236 = Unbundle By Name(w244) -> ("Accurus engaged?"=→"Accurus Engaged?":bool, "Accurus button"=→"Accurus Button":bool[], "Accurus Ch. A Vout"=→"Voltage Output Ch. A":dbl, "Accurus Ch. B Vout"=→"Voltage Output Ch. B":dbl, "Vacuum Force"=→"Vacuum Force [mmHg]" →"Vacuum Force [mmHg]  2":i32, "Irrigation engaged?"=→"Irrigation Engaged?" →"Irrigation Engaged? 2":bool)
          }
          frame Enabled {
          }
        }
        n237 = global read "Global Variables.vi" "Stage cmd Posit"() -> (w212:dbl[])
        n238 = global read "Global Variables.vi" "Stage out Posit"() -> (w213:dbl[])
        n239 = Index Array(array=w213, index #1=0 ("index"), index #2=1 ("index"), index #3=2 ("index")) -> (element #1=→"X Stage out [mm]" →"X Stage out [mm] 2":dbl, element #2=→"Y Stage out [mm]" →"Y Stage out [mm] 2":dbl, element #3=→"Z Stage out [mm]" →"Z Stage out [mm] 2":dbl)
        n240 = Index Array(array=w212, index #1=0 ("index"), index #2=1 ("index"), index #3=2 ("index")) -> (element #1=→"X Stage cmd [mm]":dbl, element #2=→"Y Stage cmd [mm]":dbl, element #3=→"Z Stage cmd [mm]":dbl)  [unwired: 1 in, 1 out]
        n241 = shared-variable "PXI-Robot\\JointAngles.lvlib\\RemoteSenderEngaged"() -> (→"Remote sender engaged":bool)  [unwired: 1 in, 1 out]
        n242 = shared-variable "PXI-Robot\\JointAngles.lvlib\\EmergencyAlarmBit"() -> (→"Emergency alarm":bool)  [unwired: 1 in, 1 out]
        n243 = global read "Global Variables.vi" "state flag array"() -> (→"State Flag Array":bool[])
        n244 = global read "Global Variables.vi" "state changing"() -> (→"State changing":bool)
        n245 = global read "Global Variables.vi" "OCT Z cmd Posit"() -> (→"OCT Z cmd [mm]":dbl)
        n246 = global read "Global Variables.vi" "OCT Z out Posit"() -> (→"OCT Z out [mm]":dbl)
        n247 = global read "Global Variables.vi" "current run no."() -> (→"Current Iter. No.":u8)
        n248 = global read "Global Variables.vi" "finished late counts"() -> (→"Finished Late Counts":u16)
        n249 = local read "Target IOP"() -> (w196:sgl)
        n250 = local read "Vac Cmd"() -> (w197:sgl)
        n251 = global read "Global Variables.vi" "pressure sensors"() -> (w194:sgl[])
        n252 = Index Array(array=w194, index=2) -> (element=w192:sgl)
        "AC Pressure [mmHg]" <- w192
        n253 = Build Array(w196, w192, w197) -> (w195:sgl[])
        n254 = Array To Cluster(array=w195) -> (cluster=→"IOP Ctrl":T7)
        n255 = Array To Cluster(array=w194) -> (cluster=→"Pressure Sensors":T8)
        n256 = case shown="True" "Clear Charts" {
          frame False {
          }
          frame True {
            w245 = T17 [] ("History Data")
            n257 = property on="IOP Ctrl" class="WFChart (strict)"("History Data"=w245) -> ()  [unwired: 2 in, 2 out]
            n258 = property on="Pressure Sensors" class="WFChart (strict)"("History Data"=w245) -> ()  [unwired: 2 in, 2 out]
          }
        }
        n259 = local read "Program Stop"() -> (w218:bool)
      }
      n260 = while {
        tunnel: w39 -> [w254]
        tunnel: w37 -> [w253]
        tunnel: [w252] -> w35
        tunnel: [w251] -> w36
        shift-right: [w249] -> _
        shift-left: T10 {"Prev L1 to L4 Posit"=[0.0, 0.0, 0.0, 0.0], "Prev Stage Posit"=[6.0, 6.0, 6.0], "Prev OCT Z Posit"=0.0} ("Prev Posit Cluster") -> [w250]
        shift-right: [w247] -> _
        shift-left: T2 {"Traj Px Array"=[], "Traj Py Array"=[], "Traj Pz Array"=[]} ("Trajectory Cluster") -> [w246]
        stop <- w248 stop-if-true
        # "State Execution Loop"
        n261 = local read "Current System State"() -> (w255:T6)
        n262 = Wait (ms)(milliseconds to wait=u32 1) -> ()  [unwired: 1 out]
        n263 = case shown="\"Tracking\"" w255 {
          tunnel: w254 -> [w269 w282 w301 w336 w372 w386 w393 w415]
          tunnel: w253 -> [w268 w281 w297 w332 w371 w385 w396 w412]
          tunnel: [w267 w280 w309 w339 w370 w384 w392 w414] -> w252
          tunnel: [w266 w279 w308 w343 w369 w383 w390 w413] -> w251
          tunnel: w250 -> [_ w278 w298 w334 w367 w382 w394 w417]
          tunnel: [w265 w277 w307 w342 w368 w381 w391 w416] -> w249
          tunnel: [w257 T2 {"Traj Px Array"=[], "Traj Py Array"=[], "Traj Pz Array"=[]} ("Trajectory Cluster") T2 {"Traj Px Array"=[], "Traj Py Array"=[], "Traj Pz Array"=[]} ("Trajectory Cluster") w337 w360 w375 w387 w410] -> w247
          tunnel: w246 -> [_ _ _ _ w360 w375 _ w410]
          frame "Homing", Default {
            w257 = T2 {"Traj Px Array"=[], "Traj Py Array"=[], "Traj Pz Array"=[]}  # Trajectory Cluster
            (unwired) 0 ("Last Index")
            n264 = local read "Offset Home 2 RCM"() -> (w264:dbl[])
            n265 = local read "Stage PID Cluster"() -> (w261:T3)
            n266 = local read "L1 to L4 PID Cluster"() -> (w262:T4)
            n267 = call "Homing.vi"("Offset Home 2 RCM"=w264, "error in"=w268, "Stage PID Cluster"=w261, "L1 to L4 PID Cluster"=w262, "FPGA VI Reference In"=w269) -> ("error out"=w266:errorcluster, "Last Stage Posit"=w258:dbl[], "Last L1 to L4 Posit"=w259:dbl[], "FPGA VI Reference Out"=w267:refnum<k20>)  [unwired: 3 in]
            n268 = Bundle By Name(cluster=T10 {"Prev L1 to L4 Posit"=[-0.5409, 0.04404050915429177, -1.917656453185038, 0.02068014705882353], "Prev Stage Posit"=[6.001471972029684, 5.996134588585126, 6.000298217087839], "Prev OCT Z Posit"=-0.0} ("Prev Posit Cluster"), "Prev L1 to L4 Posit"=w259, "Prev Stage Posit"=w258, "Prev OCT Z Posit"=0.0) -> (w265:T10)
          }
          frame "M/S Initialization" {
            n269 = local read "Offset Home 2 RCM"() -> (w271:dbl[])
            n270 = local read "Stage PID Cluster"() -> (w276:T3)
            n271 = local read "L1 to L4 PID Cluster"() -> (w275:T4)
            n272 = local read "OCT Z PID Gains"() -> (w274:cluster{"Kp":dbl, "Kd":dbl, "Ki":dbl})
            n273 = Bundle By Name(cluster=T14 {"L1 to L4 PID Cluster"={"L1 PID Gains"={"Kp"=0.005, "Kd"=0.5, "Ki"=0.0005}, "L2 PID Gains"={"Kp"=0.01, "Kd"=1.0, "Ki"=0.005}, "L3 PID Gains"={"Kp"=0.05, "Kd"=1.0, "Ki"=0.0005}, "L4 PID Gains"={"Kp"=0.1, "Kd"=0.1, "Ki"=0.0005}}, "Stage PID Cluster"={"Stage Z PID"={"Kp"=0.0005, "Kd"=0.001, "Ki"=0.0}, "Stage Y PID"={"Kp"=0.0003, "Kd"=0.01, "Ki"=0.0}, "Stage X PID"={"Kp"=0.0003, "Kd"=0.01, "Ki"=0.0}}, "OCT Z PID Gains"={"Kp"=0.0003, "Kd"=0.0001, "Ki"=0.01}} ("PID Cluster"), "Stage PID Cluster"=w276, "L1 to L4 PID Cluster"=w275, "OCT Z PID Gains"=w274) -> (w272:T14)
            n274 = call "MS Initialization v2.vi"("PID Cluster"=w272, "error in"=w281, "Offset Home 2 RCM"=w271, "Prev Posit Cluster"=w278, "FPGA VI Reference In"=w282) -> ("error out"=w279:errorcluster, "Last Posit Cluster"=w277:T18, "FPGA VI Reference Out"=w280:refnum<k20>)  [unwired: 4 in]
          }
          frame "M/S Operation" {
            (unwired) 0 ("Last Index")
            # "MS Operation"
            n275 = local read "Stage PID Cluster"() -> (w306:T3)
            n276 = local read "L1 to L4 PID Cluster"() -> (w305:T4)
            n277 = local read "OCT Z PID Gains"() -> (w304:cluster{"Kp":dbl, "Kd":dbl, "Ki":dbl})
            n278 = local read "Offset Home 2 RCM"() -> (w294:dbl[])
            n279 = local read "RUY Cluster"() -> (w287:T1)
            n280 = Bundle By Name(cluster=T14 {"L1 to L4 PID Cluster"={"L1 PID Gains"={"Kp"=0.005, "Kd"=0.5, "Ki"=0.0005}, "L2 PID Gains"={"Kp"=0.01, "Kd"=1.0, "Ki"=0.005}, "L3 PID Gains"={"Kp"=0.05, "Kd"=1.0, "Ki"=0.0005}, "L4 PID Gains"={"Kp"=0.1, "Kd"=0.1, "Ki"=0.0005}}, "Stage PID Cluster"={"Stage Z PID"={"Kp"=0.0005, "Kd"=0.001, "Ki"=0.0}, "Stage Y PID"={"Kp"=0.0003, "Kd"=0.01, "Ki"=0.0}, "Stage X PID"={"Kp"=0.0003, "Kd"=0.01, "Ki"=0.0}}, "OCT Z PID Gains"={"Kp"=0.0003, "Kd"=0.0001, "Ki"=0.01}} ("PID Cluster"), "Stage PID Cluster"=w306, "L1 to L4 PID Cluster"=w305, "OCT Z PID Gains"=w304) -> (w283:T14)
            n281 = global read "Global Variables.vi" "current iter. no."() -> (w285:u16)
            n282 = feedback #1() -> (w286:u16)  [unwired: 1 in]
            n283 = feedback-in #1(w285) -> ()
            n284 = Not Equal?(x=w285, y=w286) -> (x != y?=w284:bool)
            n285 = flat-sequence {
              tunnel: w301 -> [w319]
              tunnel: w298 -> [w318]
              tunnel: w297 -> [w317]
              tunnel: w294 -> [w316]
              tunnel: w283 -> [w315]
              tunnel: [w319] -> w292
              tunnel: [w318] -> w291
              tunnel: [w317] -> w290
              tunnel: [w316] -> w289
              tunnel: [w315] -> w288
              tunnel: w287 -> [w314]
              tunnel: w284 -> [_]
              tunnel: [w321] -> w293
              tunnel: [w322] -> w295
              tunnel: [w323] -> w296
              tunnel: [w324] -> w299
              tunnel: [w325] -> w300
              tunnel: w292 -> [w325]
              tunnel: w291 -> [w324]
              tunnel: w290 -> [w323]
              tunnel: w289 -> [w322]
              tunnel: w288 -> [w321]
              frame #0 {
                # "Plot ILC results"
                n286 = Unbundle By Name(w314) -> ("uFF.theta 1 Array"=→"L1 Cmd":dbl[], "uFF.theta 2 Array"=→"L2 Cmd":dbl[], "uFF.d3 Array"=→"L3 Cmd":dbl[], "uFF.theta 4 Array"=→"L4 Cmd":dbl[])
              }
              frame #1 {
                n287 = global write "Global Variables.vi" "plotting finished"(TRUE ("state changing")) -> ()
              }
            }
            n288 = call "MS Operation IOP Ctrl v2.vi"("PID Cluster"=w293, "error in"=w296, "Offset Home 2 RCM"=w295, "Prev Posit Cluster"=w299, "FPGA VI Reference In"=w300) -> ("error out"=w308:errorcluster, "Last Posit Cluster"=w307:T18, "FPGA VI Reference Out"=w309:refnum<k20>)  [unwired: 4 in]
          }
          frame "Trajectory Loading" {
            n289 = local read "Offset Home 2 RCM"() -> (w333:dbl[])
            n290 = local read "Stage PID Cluster"() -> (w348:T3)
            n291 = local read "L1 to L4 PID Cluster"() -> (w347:T4)
            n292 = local read "OCT Z PID Gains"() -> (w346:cluster{"Kp":dbl, "Kd":dbl, "Ki":dbl})
            n293 = Bundle By Name(cluster=T14 {"L1 to L4 PID Cluster"={"L1 PID Gains"={"Kp"=0.005, "Kd"=0.5, "Ki"=0.0005}, "L2 PID Gains"={"Kp"=0.01, "Kd"=1.0, "Ki"=0.005}, "L3 PID Gains"={"Kp"=0.05, "Kd"=1.0, "Ki"=0.0005}, "L4 PID Gains"={"Kp"=0.1, "Kd"=0.1, "Ki"=0.0005}}, "Stage PID Cluster"={"Stage Z PID"={"Kp"=0.0005, "Kd"=0.001, "Ki"=0.0}, "Stage Y PID"={"Kp"=0.0003, "Kd"=0.01, "Ki"=0.0}, "Stage X PID"={"Kp"=0.0003, "Kd"=0.01, "Ki"=0.0}}, "OCT Z PID Gains"={"Kp"=0.0003, "Kd"=0.0001, "Ki"=0.01}} ("PID Cluster"), "Stage PID Cluster"=w348, "L1 to L4 PID Cluster"=w347, "OCT Z PID Gains"=w346) -> (w331:T14)
            n294 = call "Trajectory Loading Polishing.vi"("PID Cluster"=w331, "error in"=w332, "Offset Home 2 RCM"=w333, "Prev Posit Cluster"=w334, "FPGA VI Reference In"=w336) -> ("RUY Cluster"=w329:T1, "Trajectory Cluster"=w328:T2, "Last Posit Cluster"=w327:T18, "FPGA VI Reference Out"=w326:refnum<k20>, "error out"=w330:errorcluster, "First Trk Pt"=→"First Trk Pt":dbl[])  [unwired: 1 in]
            n295 = flat-sequence {
              tunnel: w328 -> [w354]
              tunnel: w330 -> [w353]
              tunnel: [w353] -> w344
              tunnel: w327 -> [w352]
              tunnel: [w352] -> w341
              tunnel: w326 -> [w351]
              tunnel: [w351] -> w340
              tunnel: [w350] -> w338
              tunnel: w328 -> [w350]
              tunnel: w329 -> [w349]
              tunnel: [w358] -> w343
              tunnel: w344 -> [w358]
              tunnel: [w357] -> w342
              tunnel: w341 -> [w357]
              tunnel: w340 -> [w356]
              tunnel: [w356] -> w339
              tunnel: w338 -> [w355]
              tunnel: [w355] -> w337
              frame #0 {
                n296 = local write "RUY Cluster"(w349) -> ()
                "Trajectory Cluster" <- w354
              }
              frame #1 {
                "Update Mdl & Traj" <- TRUE
              }
            }
          }
          frame "Tracking Initialization" {
            n297 = local read "Stage PID Cluster"() -> (w365:T3)
            n298 = local read "L1 to L4 PID Cluster"() -> (w364:T4)
            n299 = local read "OCT Z PID Gains"() -> (w362:cluster{"Kp":dbl, "Kd":dbl, "Ki":dbl})
            n300 = local read "Offset Home 2 RCM"() -> (w366:dbl[])
            n301 = Bundle By Name(cluster=T14 {"L1 to L4 PID Cluster"={"L1 PID Gains"={"Kp"=0.005, "Kd"=0.5, "Ki"=0.0005}, "L2 PID Gains"={"Kp"=0.01, "Kd"=1.0, "Ki"=0.005}, "L3 PID Gains"={"Kp"=0.05, "Kd"=1.0, "Ki"=0.0005}, "L4 PID Gains"={"Kp"=0.1, "Kd"=0.1, "Ki"=0.0005}}, "Stage PID Cluster"={"Stage Z PID"={"Kp"=0.0005, "Kd"=0.001, "Ki"=0.0}, "Stage Y PID"={"Kp"=0.0003, "Kd"=0.01, "Ki"=0.0}, "Stage X PID"={"Kp"=0.0003, "Kd"=0.01, "Ki"=0.0}}, "OCT Z PID Gains"={"Kp"=0.0003, "Kd"=0.0001, "Ki"=0.01}} ("PID Cluster"), "Stage PID Cluster"=w365, "L1 to L4 PID Cluster"=w364, "OCT Z PID Gains"=w362) -> (w361:T14)
            n302 = call "Tracking Initialization v2.vi"("Trajectory Cluster"=w360, "PID Cluster"=w361, "Offset Home 2 RCM"=w366, "error in"=w371, "Prev Posit Cluster"=w367, "FPGA VI Reference In"=w372) -> ("error out"=w369:errorcluster, "Last Posit Cluster"=w368:T18, "FPGA VI Reference Out"=w370:refnum<k20>)  [unwired: 3 in]
          }
          frame "Tracking" {
            n303 = local read "Stage PID Cluster"() -> (w380:T3)
            n304 = local read "L1 to L4 PID Cluster"() -> (w379:T4)
            n305 = local read "OCT Z PID Gains"() -> (w378:cluster{"Kp":dbl, "Kd":dbl, "Ki":dbl})
            n306 = local read "Offset Home 2 RCM"() -> (w374:dbl[])
            n307 = Bundle By Name(cluster=T14 {"L1 to L4 PID Cluster"={"L1 PID Gains"={"Kp"=0.005, "Kd"=0.5, "Ki"=0.0005}, "L2 PID Gains"={"Kp"=0.01, "Kd"=1.0, "Ki"=0.005}, "L3 PID Gains"={"Kp"=0.05, "Kd"=1.0, "Ki"=0.0005}, "L4 PID Gains"={"Kp"=0.1, "Kd"=0.1, "Ki"=0.0005}}, "Stage PID Cluster"={"Stage Z PID"={"Kp"=0.0005, "Kd"=0.001, "Ki"=0.0}, "Stage Y PID"={"Kp"=0.0003, "Kd"=0.01, "Ki"=0.0}, "Stage X PID"={"Kp"=0.0003, "Kd"=0.01, "Ki"=0.0}}, "OCT Z PID Gains"={"Kp"=0.0003, "Kd"=0.0001, "Ki"=0.01}} ("PID Cluster"), "Stage PID Cluster"=w380, "L1 to L4 PID Cluster"=w379, "OCT Z PID Gains"=w378) -> (w376:T14)
            n308 = local read "No. Cycles"() -> (w373:u8)
            n309 = call "Tracking v2.vi"("Offset Home 2 RCM"=w374, "Trajectory Cluster"=w375, "PID Cluster"=w376, "No. Cycles"=w373, "error in"=w385, "Prev Posit Cluster"=w382, "FPGA VI Reference In"=w386) -> ("error out"=w383:errorcluster, "Last Posit Cluster"=w381:T18, "FPGA VI Reference Out"=w384:refnum<k20>)  [unwired: 2 in]
            n310 = disable-structure shown="Disabled" {
              frame Disabled {
                n311 = local read "RUY Cluster"() -> ()  [unwired: 1 in]
              }
              frame Enabled {
              }
            }
          }
          frame "Physical Learning" {
            n312 = local read "Offset Home 2 RCM"() -> (w395:dbl[])
            n313 = local read "RUY Cluster"() -> (w389:T1)
            n314 = local read "L1 to L4 PID Cluster"() -> (w401:T4)
            n315 = local read "Stage PID Cluster"() -> (w400:T3)
            n316 = local read "OCT Z PID Gains"() -> (w399:cluster{"Kp":dbl, "Kd":dbl, "Ki":dbl})
            n317 = Bundle By Name(cluster=T14 {"L1 to L4 PID Cluster"={"L1 PID Gains"={"Kp"=0.005, "Kd"=0.5, "Ki"=0.0005}, "L2 PID Gains"={"Kp"=0.01, "Kd"=1.0, "Ki"=0.005}, "L3 PID Gains"={"Kp"=0.05, "Kd"=1.0, "Ki"=0.0005}, "L4 PID Gains"={"Kp"=0.1, "Kd"=0.1, "Ki"=0.0005}}, "Stage PID Cluster"={"Stage Z PID"={"Kp"=0.0005, "Kd"=0.001, "Ki"=0.0}, "Stage Y PID"={"Kp"=0.0003, "Kd"=0.01, "Ki"=0.0}, "Stage X PID"={"Kp"=0.0003, "Kd"=0.01, "Ki"=0.0}}, "OCT Z PID Gains"={"Kp"=0.0003, "Kd"=0.0001, "Ki"=0.01}} ("PID Cluster"), "Stage PID Cluster"=w400, "L1 to L4 PID Cluster"=w401, "OCT Z PID Gains"=w399) -> (w398:T14)
            n318 = local read "Learning Gains"() -> (w397:dbl[])
            n319 = call "Physical Learning v2.vi"("Learning Gains"=w397, "PID Cluster"=w398, "Input RUY"=w389, "error in"=w396, "Offset Home 2 RCM"=w395, "Prev Posit Cluster"=w394, "FPGA VI Reference In"=w393) -> ("error out"=w390:errorcluster, "Updated Trajectory"=w387:T2, "Last Posit Cluster"=w391:T18, "FPGA VI Reference Out"=w392:refnum<k20>, "Updated RUY"=w388:T1)
            n320 = local write "RUY Cluster"(w388) -> ()
          }
          frame "Cyber Learning" {
            n321 = local read "Offset Home 2 RCM"() -> (w409:dbl[])
            n322 = local read "L1 to L4 PID Cluster"() -> (w405:T4)
            n323 = local read "Stage PID Cluster"() -> (w406:T3)
            n324 = local read "OCT Z PID Gains"() -> (w404:cluster{"Kp":dbl, "Kd":dbl, "Ki":dbl})
            n325 = local read "RUY Cluster"() -> (w411:T1)
            n326 = Bundle By Name(cluster=T14 {"L1 to L4 PID Cluster"={"L1 PID Gains"={"Kp"=0.005, "Kd"=0.5, "Ki"=0.0005}, "L2 PID Gains"={"Kp"=0.01, "Kd"=1.0, "Ki"=0.005}, "L3 PID Gains"={"Kp"=0.05, "Kd"=1.0, "Ki"=0.0005}, "L4 PID Gains"={"Kp"=0.1, "Kd"=0.1, "Ki"=0.0005}}, "Stage PID Cluster"={"Stage Z PID"={"Kp"=0.0005, "Kd"=0.001, "Ki"=0.0}, "Stage Y PID"={"Kp"=0.0003, "Kd"=0.01, "Ki"=0.0}, "Stage X PID"={"Kp"=0.0003, "Kd"=0.01, "Ki"=0.0}}, "OCT Z PID Gains"={"Kp"=0.0003, "Kd"=0.0001, "Ki"=0.01}} ("PID Cluster"), "Stage PID Cluster"=w406, "L1 to L4 PID Cluster"=w405, "OCT Z PID Gains"=w404) -> (w407:T14)
            n327 = call "ILC Cyber Learning.vi"("PID Cluster"=w407, "Input RUY"=w411, "error in"=w412, "Offset Home 2 RCM"=w409, "Prev Posit Cluster"=w417, "FPGA VI Reference In"=w415) -> ("error out"=w413:errorcluster, "Last Posit Cluster"=w416:T18, "FPGA VI Reference Out"=w414:refnum<k20>, "Updated RUY"=w403:T1)  [unwired: 2 in]
            n328 = local write "RUY Cluster"(w403) -> ()
          }
        }
        n329 = local read "Program Stop"() -> (w248:bool)
      }
      n330 = while {
        stop <- w45 stop-if-true
        # "IOP Data Logging"
        n331 = flat-sequence {
          tunnel: [w49] -> w48
          tunnel: [w51] -> w47
          tunnel: [w50] -> w46
          tunnel: w48 -> [w70]
          tunnel: w47 -> [w69]
          tunnel: w46 -> [w68]
          frame #0 {
            n332 = while {
              tunnel: [w66] -> w51
              tunnel: [w61] -> w50
              tunnel: [w65] -> w49
              stop <- w67 stop-if-true
              n333 = Wait (ms)(milliseconds to wait=u32 100) -> ()  [unwired: 1 out]
              n334 = Number To Fractional String(number="Data No", precision (6)=i16 0) -> (F-format string=w52:string)  [unwired: 2 in]
              n335 = Concatenate Strings("C:\\IOPData", w52, ".txt" ("string")) -> (w54:string)
              n336 = shared-variable "PXI-Robot\\JointAngles.lvlib\\Data No"(w52) -> ()  [unwired: 1 in, 1 out]
              n337 = local read "Program Stop"() -> (w63:bool)
              n338 = local read "Take IOP Data"() -> (w60:bool)
              n339 = String To Path(string=w54) -> (path=w53:path)
              "File Path" <- w53
              n340 = call <vilib>:"Check if File or Folder Exists.vi"("path"=w53) -> ("file or folder exists?"=w62:bool, "dup path"=w66:path)  [unwired: 8 in, 1 out]
              "File Exists" <- w62
              n341 = Not(x=w62) -> (.not. x?=w59:bool)
              n342 = shared-variable "PXI-Robot\\JointAngles.lvlib\\Save Data"(w60) -> ()  [unwired: 1 in, 1 out]
              n343 = global read "Global Variables.vi" "seconds of data"() -> (w61:sgl)
              n344 = And(x=w60, y=w59) -> (x .and. y?=w65:bool)
              n345 = Compound Arithmetic op=OR(w63, w65) -> (w67:bool)
            }
          }
          frame #1 {
            n346 = case shown="True" w70 {
              tunnel: w69 -> [_ w75]
              tunnel: w68 -> [_ w72]
              frame False {
              }
              frame True {
                n347 = flat-sequence {
                  tunnel: w75 -> [w86]
                  tunnel: [w84] -> w74
                  tunnel: [w80] -> w73
                  tunnel: w72 -> [w94]
                  tunnel: [w92] -> w71
                  tunnel: w74 -> [w99]
                  tunnel: w73 -> [w98]
                  tunnel: w71 -> [w97]
                  frame #0 {
                    w80 = 10  # Period: 10 [ms]
                    n348 = Build Array("t" ("delimiter (\\t)"), "Pdes" ("delimiter (\\t)"), "Vcmd" ("delimiter (\\t)"), "Pirr" ("delimiter (\\t)"), "Pvac" ("delimiter (\\t)"), "Pac" ("delimiter (\\t)"), "Pvit" ("delimiter (\\t)"), "X" ("delimiter (\\t)"), "Y" ("delimiter (\\t)"), "Z" ("delimiter (\\t)"), "OCT" ("delimiter (\\t)")) -> (w83:string[])
                    n349 = call-poly <vilib>:"Write Delimited Spreadsheet.vi"("file path (dialog if empty)"=w86, "format (%s)"="%s", "1D data"=w83, "delimiter (\\t)"="," ("delimiter (\\t)")) -> ("new file path (Not A Path if cancelled)"=w84:path)  [unwired: 10 in, 1 out]
                    n350 = Multiply(x=w80, y=0.001) -> (x*y=w93:dbl)
                    n351 = Divide(x=w94, y=w93) -> (x/y=w92:dbl)
                  }
                  frame #1 {
                    n352 = while {
                      tunnel: w99 -> [w116]
                      tunnel: w98 -> [w119]
                      tunnel: w97 -> [w117]
                      i -> [w118]
                      stop <- w121 stop-if-true
                      n353 = Wait (ms)(milliseconds to wait=w119) -> ()  [unwired: 1 out]
                      n354 = Greater Or Equal?(x=w118, y=w117) -> (x >= y?=w105:bool)
                      n355 = local read "Target IOP"() -> (w112:sgl)
                      n356 = local read "Vac Cmd"() -> (w111:sgl)
                      n357 = local read "Pressure Reading"() -> (w110:dbl[])
                      n358 = local read "Tip out Posit"() -> (w107:dbl[])
                      n359 = local read "OCT Z out [mm]"() -> (w108:dbl)
                      n360 = local read "Program Stop"() -> (w109:bool)
                      n361 = Compound Arithmetic op=MULTIPLY(w118, w119, 0.001 ("y")) -> (w100:dbl)
                      "Elaspsed Time" <- w100
                      n362 = Not(x=w105) -> (.not. x?=w106:bool)
                      n363 = shared-variable "PXI-Robot\\JointAngles.lvlib\\Save Data"(w106) -> ()  [unwired: 1 in, 1 out]
                      n364 = Compound Arithmetic op=OR(w109, w105) -> (w121:bool)
                      n365 = Build Array (concatenate)(w100, w112, w111, w110, w107, w108) -> (w114:dbl[])
                      n366 = call-poly <vilib>:"Write Delimited Spreadsheet.vi"("file path (dialog if empty)"=w116, "1D data"=w114, "append to file? (new file:F)"=TRUE, "delimiter (\\t)"="," ("delimiter (\\t)")) -> ()  [unwired: 10 in, 2 out]
                      n367 = Multiply(x=w100, y=100.0) -> (x*y=w102:dbl)
                      n368 = Format Into String(format string="%06d", w102) -> (resulting string=w103:string)  [unwired: 2 in, 1 out]
                      n369 = shared-variable "PXI-Robot\\JointAngles.lvlib\\TimeStamp"(w103) -> ()  [unwired: 1 in, 1 out]
                    }
                  }
                }
              }
            }
          }
          frame #2 {
            n370 = local write "Take IOP Data"(FALSE) -> ()
          }
        }
        n371 = local read "Program Stop"() -> (w45:bool)
      }
      n372 = node-c288(w43) -> ()  [unwired: 1 out]
    }
    frame #2 {
      n373 = while {
        shift-right: [w619] -> w611
        shift-left: w609 -> [w621]
        shift-right: [w618] -> w610
        shift-left: w608 -> [w620]
        stop <- w612 stop-if-true
        w616 = 0.0 ("OCT  Z cmd Posit [mm]")
        # "Move OCT back to 0"
        n374 = call "OCT Reference Follower.vi"("OCT  Z cmd Posit [mm]"=w616, "error in"=w620, "FPGA VI Reference In"=w621) -> ("OCT  Z out Posit [mm]"=w617:dbl, "error out"=w618:errorcluster, "FPGA VI Reference Out"=w619:refnum<k20>)  [unwired: 6 in]
        n375 = Subtract(x=w617, y=w616) -> (x-y=w615:dbl)
        n376 = Absolute Value(x=w615) -> (abs(x)=w614:dbl)
        n377 = Less?(x=w614, y=0.1) -> (x < y?=w612:bool)
      }
    }
    frame #3 {
      w626 = FALSE
      w628 = i16 0 ("element")
      n378 = Build Array(w628, w628, w628, w628, w628, w628, w628, w628) -> (w627:i16[])
      n379 = xnode "Output Shut Down"("FPGA VI Reference In"=w623, "error in"=w622, "AO"=w627, "INHB X"=w626, "INHB Y"=w626, "INHB Z"=w626, "INHB OCT Mot"=w626) -> ("FPGA VI Reference Out"=w625:refnum<k20>, "error out"=w624:errorcluster)
    }
    frame #4 {
      # "Close Applicaion"
      n380 = xnode "FPGA Reset"("FPGA VI Reference In"=w630, "error in"=w629) -> ("FPGA VI Reference Out"=w633:refnum<k20>, "error out"=w632:errorcluster)
      n381 = xnode "Close FPGA VI Reference"("FPGA VI Reference In"=w633, "error in"=w632) -> ("error out"=→"Error(s) Out on Program End":errorcluster)
    }
  }
